vi "cDAQ Cal UI.vi"(11 "Calling VI Ref":refnum<vi>) -> ()   [LabVIEW 2013]
uses:
  Type Defs/Units Type Def (DAQ Rack).ctl
  Type Defs/cDAQ Type Def (cDAQ).ctl
  Type Defs/Rack Version Type Def.ctl
  Type Defs/Registered System.ctl
  Type Defs/System Type.ctl
  Type Defs/cDAQ Targets Type Def.ctl
  Type Defs/Target Cluster Type Def.ctl
  Type Defs/Setpoint Cluster Type Def.ctl
  Type Defs/TCP Data Stream Mode (PC).ctl
  <vilib>/Utility/miscctls.llb/LVRowAndColumnTypeDef.ctl
  <vilib>/Utility/file.llb/Write To Spreadsheet File (string).vi
  <vilib>/Utility/file.llb/Read From Spreadsheet File (string).vi
  <userlib>/_OpenG.lib/array/array.llb/Remove Duplicates from 1D Array (DBL)__ogtk.vi
  <userlib>/_OpenG.lib/array/array.llb/Search 1D Array (String)__ogtk.vi
  <vilib>/ptbypt/NI_PtbyPt.lvlib
  <vilib>/Analysis/NI_AALPro.lvlib
  <vilib>/Utility/config.llb/NI_LVConfig.lvlib
  <vilib>/FTP/NI_FTP.lvlib
panel:
  out "RIO Found":bool
  out "Lost Connection":bool
  in  "Stop Second Loop":bool
  out "a0":dbl format="%#.4g"
  out "a2":dbl format="%#.4g"
  out "a1":dbl format="%#.4g"
  out "a3":dbl format="%#.4g"
  out "a4":dbl format="%#.4g"
  in  "App Dir":path
  in  "Load Indicator Tab":enum32{"Page 1"}(tab)
  in  "Header Tab":enum32{"Page 1", "Page 2"}(tab)
  in  "Header OK":bool
  in  "Header Cancel":bool
  in  "Header Comments":string[][](table)=[[""], [""], [""]]
  in  "Cal Standards Table":string[][](table)=[["", ""], ["", ""], ["", ""], ["", ""], ["", ""]]
  in  "Sys Cal Table":string[][](table)=[["", ""], ["", ""], ["", ""], ["", ""], ["", ""]]
  in  "Header Table 1":string[][](table)=[[""], [""], [""], [""], [""], [""], [""], [""]]
  in  "Header Table 2":string[][](table)=[[""], [""], [""], [""], [""], [""], [""]]
  in  "debug":bool=TRUE
  in  "Output Tab":enum32{"Page 1", "Page 2"}(tab)
  out "Row":i32
  in  "Main Tab":enum32{"Page 1", "Page 2"}(tab)
  in  "Transfer Cal":bool
  in  "Verify Tab":enum32{"Page 1", "Page 2"}(tab)
  out "Ver Reading":dbl=0.0016 caption="reading" format="%#.4g"
  in  "Hide Devs":bool
  in  "Auto":bool
  in  "Hide Cal Values":bool
  in  "Verify Edit":bool
  in  "Verify Table":string[][](table)=[["", "0", "0"], ["", "3", "3"], ["", "6", "6"], ["", "9", "9"], ["", "12", "12"], ["", "15", "15"], ["", "", ""], ["", "", ""], ["", "", ""], ["", "", ""]]
  in  "Verify Read":bool
  in  "ms":u32=1000
  in  "avg":i32=5
  in  "Save Cal":bool
  in  "Cancel Verify":bool
  in  "Cal Tab":enum32{"Apply", "Cal"}(tab)
  in  "Cancel Cal":bool
  in  "Apply Cal":bool
  in  "Confirm Cal Point":bool
  in  "Master Value":dbl caption="cal pt" format="%#.4g"
  out "Cal Reading":dbl=0.0016 caption="reading" format="%#.4g"
  in  "4th Point Cal":bool
  out "Reading Value 4":dbl caption="reading" format="%#.4g"
  in  "Cal Value 4":dbl caption="cal pt" format="%#.4g"
  in  "5th Point Cal":bool
  out "Reading Value 5":dbl caption="reading" format="%#.4g"
  in  "Cal Value 5":dbl caption="cal pt" format="%#.4g"
  in  "Start Verification":bool
  in  "Header":bool
  out "Cal Table":string[][](table)=[["AI-00", "V", "", "", "", "", "", "", "", "", "", "", "", "", "", "", "", "", "", "", "", "", "", "", "", "", "", "", "", "", "", ""], ["AI-01", "V", "", "", "", "", "", "", "", "", "", "", "", "", "", "", "", "", "", "", "", "", "", "", "", "", "", "", "", "", "", ""], ["AI-02", "V", "", "", "", "", "", "", "", "", "", "", "", "", "", "", "", "", "", "", "", "", "", "", "", "", "", "", "", "", "", ""], ["AI-03", "V", "", "", "", "", "", "", "", "", "", "", "", "", "", "", "", "", "", "", "", "", "", "", "", "", "", "", "", "", "", ""], ["AI-04", "V", "", "", "", "", "", "", "", "", "", "", "", "", "", "", "", "", "", "", "", "", "", "", "", "", "", "", "", "", "", ""], ["AI-05", "V", "", "", "", "", "", "", "", "", "", "", "", "", "", "", "", "", "", "", "", "", "", "", "", "", "", "", "", "", "", ""], ["AI-06", "V", "", "", "", "", "", "", "", "", "", "", "", "", "", "", "", "", "", "", "", "", "", "", "", "", "", "", "", "", "", ""], ["AI-07", "V", "", "", "", "", "", "", "", "", "", "", "", "", "", "", "", "", "", "", "", "", "", "", "", "", "", "", "", "", "", ""], ["AI-08", "V", "", "", "", "", "", "", "", "", "", "", "", "", "", "", "", "", "", "", "", "", "", "", "", "", "", "", "", "", "", ""], ["AI-09", "V", "", "", "", "", "", "", "", "", "", "", "", "", "", "", "", "", "", "", "", "", "", "", "", "", "", "", "", "", "", ""], ["AI-10", "V", "", "", "", "", "", "", "", "", "", "", "", "", "", "", "", "", "", "", "", "", "", "", "", "", "", "", "", "", "", ""], ["AI-11", "V", "", "", "", "", "", "", "", "", "", "", "", "", "", "", "", "", "", "", "", "", "", "", "", "", "", "", "", "", "", ""], ["AI-12", "V", "", "", "", "", "", "", "", "", "", "", "", "", "", "", "", "", "", "", "", "", "", "", "", "", "", "", "", "", "", ""], ["AI-13", "V", "", "", "", "", "", "", "", "", "", "", "", "", "", "", "", "", "", "", "", "", "", "", "", "", "", "", "", "", "", ""], ["AI-14", "V", "", "", "", "", "", "", "", "", "", "", "", "", "", "", "", "", "", "", "", "", "", "", "", "", "", "", "", "", "", ""], ["AI-15", "V", "", "", "", "", "", "", "", "", "", "", "", "", "", "", "", "", "", "", "", "", "", "", "", "", "", "", "", "", "", ""], ["AI-16", "V", "", "", "", "", "", "", "", "", "", "", "", "", "", "", "", "", "", "", "", "", "", "", "", "", "", "", "", "", "", ""], ["AI-17", "V", "", "", "", "", "", "", "", "", "", "", "", "", "", "", "", "", "", "", "", "", "", "", "", "", "", "", "", "", "", ""], ["AI-18", "V", "", "", "", "", "", "", "", "", "", "", "", "", "", "", "", "", "", "", "", "", "", "", "", "", "", "", "", "", "", ""], ["AI-19", "V", "", "", "", "", "", "", "", "", "", "", "", "", "", "", "", "", "", "", "", "", "", "", "", "", "", "", "", "", "", ""], ["AI-20", "V", "", "", "", "", "", "", "", "", "", "", "", "", "", "", "", "", "", "", "", "", "", "", "", "", "", "", "", "", "", ""], ["AI-21", "V", "", "", "", "", "", "", "", "", "", "", "", "", "", "", "", "", "", "", "", "", "", "", "", "", "", "", "", "", "", ""], ["AI-22", "V", "", "", "", "", "", "", "", "", "", "", "", "", "", "", "", "", "", "", "", "", "", "", "", "", "", "", "", "", "", ""], ["AI-23", "V", "", "", "", "", "", "", "", "", "", "", "", "", "", "", "", "", "", "", "", "", "", "", "", "", "", "", "", "", "", ""], ["AI-24", "V", "", "", "", "", "", "", "", "", "", "", "", "", "", "", "", "", "", "", "", "", "", "", "", "", "", "", "", "", "", ""], ["AI-25", "V", "", "", "", "", "", "", "", "", "", "", "", "", "", "", "", "", "", "", "", "", "", "", "", "", "", "", "", "", "", ""], ["AI-26", "V", "", "", "", "", "", "", "", "", "", "", "", "", "", "", "", "", "", "", "", "", "", "", "", "", "", "", "", "", "", ""], ["AI-27", "V", "", "", "", "", "", "", "", "", "", "", "", "", "", "", "", "", "", "", "", "", "", "", "", "", "", "", "", "", "", ""], ["AI-28", "V", "", "", "", "", "", "", "", "", "", "", "", "", "", "", "", "", "", "", "", "", "", "", "", "", "", "", "", "", "", ""], ["AI-29", "V", "", "", "", "", "", "", "", "", "", "", "", "", "", "", "", "", "", "", "", "", "", "", "", "", "", "", "", "", "", ""], ["AI-30", "V", "", "", "", "", "", "", "", "", "", "", "", "", "", "", "", "", "", "", "", "", "", "", "", "", "", "", "", "", "", ""], ["AI-31", "V", "", "", "", "", "", "", "", "", "", "", "", "", "", "", "", "", "", "", "", "", "", "", "", "", "", "", "", "", "", ""], ["TC-00", "degF", "", "", "", "", "", "", "", "", "", "", "", "", "", "", "", "", "", "", "", "", "", "", "", "", "", "", "", "", "", ""], ["TC-01", "degF", "", "", "", "", "", "", "", "", "", "", "", "", "", "", "", "", "", "", "", "", "", "", "", "", "", "", "", "", "", ""], ["TC-02", "degF", "", "", "", "", "", "", "", "", "", "", "", "", "", "", "", "", "", "", "", "", "", "", "", "", "", "", "", "", "", ""], ["TC-03", "degF", "", "", "", "", "", "", "", "", "", "", "", "", "", "", "", "", "", "", "", "", "", "", "", "", "", "", "", "", "", ""], ["TC-04", "degF", "", "", "", "", "", "", "", "", "", "", "", "", "", "", "", "", "", "", "", "", "", "", "", "", "", "", "", "", "", ""], ["TC-05", "degF", "", "", "", "", "", "", "", "", "", "", "", "", "", "", "", "", "", "", "", "", "", "", "", "", "", "", "", "", "", ""], ["TC-06", "degF", "", "", "", "", "", "", "", "", "", "", "", "", "", "", "", "", "", "", "", "", "", "", "", "", "", "", "", "", "", ""], ["TC-07", "degF", "", "", "", "", "", "", "", "", "", "", "", "", "", "", "", "", "", "", "", "", "", "", "", "", "", "", "", "", "", ""], ["TC-08", "degF", "", "", "", "", "", "", "", "", "", "", "", "", "", "", "", "", "", "", "", "", "", "", "", "", "", "", "", "", "", ""], ["TC-09", "degF", "", "", "", "", "", "", "", "", "", "", "", "", "", "", "", "", "", "", "", "", "", "", "", "", "", "", "", "", "", ""], ["TC-10", "degF", "", "", "", "", "", "", "", "", "", "", "", "", "", "", "", "", "", "", "", "", "", "", "", "", "", "", "", "", "", ""], ["TC-11", "degF", "", "", "", "", "", "", "", "", "", "", "", "", "", "", "", "", "", "", "", "", "", "", "", "", "", "", "", "", "", ""], ["TC-12", "degF", "", "", "", "", "", "", "", "", "", "", "", "", "", "", "", "", "", "", "", "", "", "", "", "", "", "", "", "", "", ""], ["TC-13", "degF", "", "", "", "", "", "", "", "", "", "", "", "", "", "", "", "", "", "", "", "", "", "", "", "", "", "", "", "", "", ""], ["TC-14", "degF", "", "", "", "", "", "", "", "", "", "", "", "", "", "", "", "", "", "", "", "", "", "", "", "", "", "", "", "", "", ""], ["TC-15", "degF", "", "", "", "", "", "", "", "", "", "", "", "", "", "", "", "", "", "", "", "", "", "", "", "", "", "", "", "", "", ""], ["", "", "", "", "", "", "", "", "", "", "", "", "", "", "", "", "", "", "", "", "", "", "", "", "", "", "", "", "", "", "", ""]]
  out "Tank IP:":string
  in  "Start Cal":bool
  in  "1st Point Cal":bool
  out "Reading Value 1":dbl caption="Read Data" format="%#.4g"
  in  "Cal Value 1":dbl caption="Cal Point" format="%#.4g"
  in  "2nd Point Cal":bool
  out "Reading Value 2":dbl caption="reading" format="%#.4g"
  in  "Cal Value 2":dbl caption="cal pt" format="%#.4g"
  in  "Cal Unit":T1
  in  "3rd Point Cal":bool
  out "Reading Value 3":dbl caption="reading" format="%#.4g"
  in  "Cal Value 3":dbl caption="cal pt" format="%#.4g"
  in  "View Spreadsheet":bool
  in  "Channel to Cal":T2
  # "Channel Data"
  # "System Calibration Components"
  # "Calibration Standards Used"
  # "Output Control"
  # "Enter Header Info"
  # "Calibration"
  # "Verification"
  # "Select Channel to Calibrate"
  # "Cal Spreadsheet"
  # "*Excel must be closed to return control to this app."
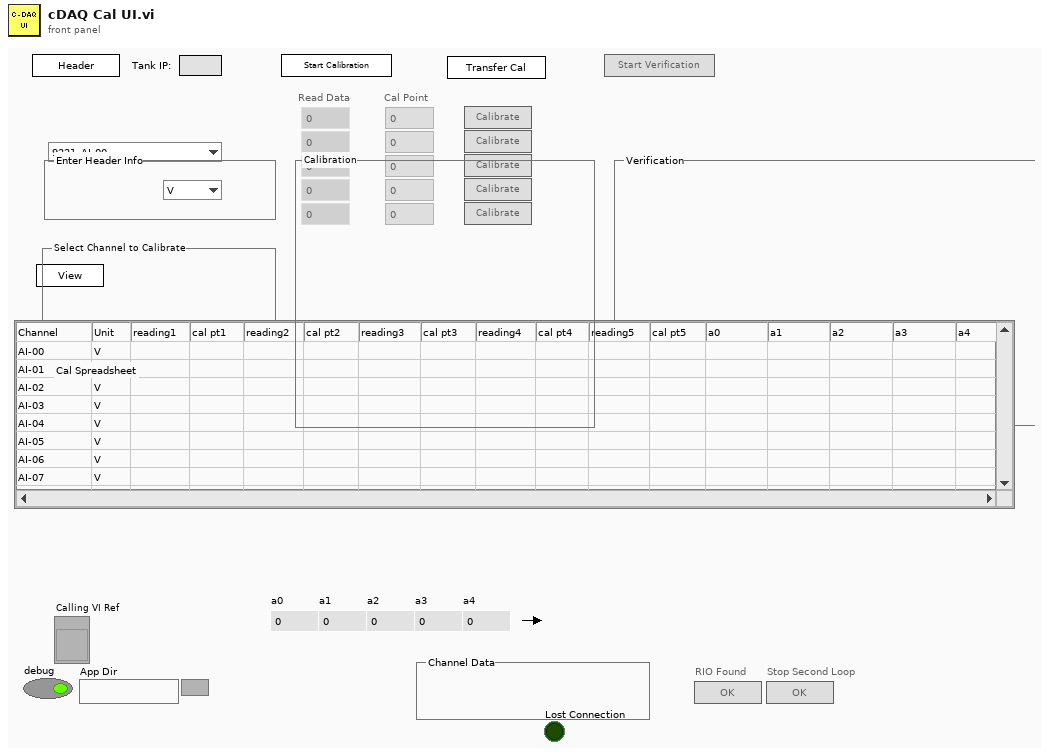
[diagram p1: front panel]
types:
  T1 = typedef "Units Type Def (DAQ Rack).ctl" = enum16{"V", "mA", "A", "Hz", "deg C"}
  T2 = typedef "cDAQ Type Def (cDAQ).ctl" = enum16{"9221_AI-00", "9221_AI-01", "9221_AI-02", "9221_AI-03", "9221_AI-04", "9221_AI-05", "9221_AI-06", "9221_AI-07", "9205_AI-00", "9205_AI-01", "9205_AI-02", "9205_AI-03", "9205_AI-04", "9205_AI-05", "9205_AI-06", "9205_AI-07", "9208_AI-00", "9208_AI-01", "9208_AI-02", "9208_AI-03", "9208_AI-04", "9208_AI-05", "9208_AI-06", "9208_AI-07", "9211_TC-00", "9211_TC-01", "9211_TC-02", "9211_TC-03"}
  T3 = typedef "cDAQ Targets Type Def.ctl" = cluster{"9221 Targets":T4, "9205 Targets":T4, "9208 Targets":T4, "9221 Setpoints":T5, "9205 Setpoints":T5, "9208 Setpoints ":T5, "9211 Targets":T4, "9211 Setpoints":T5}
  T4 = typedef "Target Cluster Type Def.ctl" = cluster{"target1":dbl, "target2":dbl, "target3":dbl, "target4":dbl, "target5":dbl, "target6":dbl, "target7":dbl, "target8":dbl, "target9":dbl, "target10":dbl}
  T5 = typedef "Setpoint Cluster Type Def.ctl" = cluster{"setpoint1":dbl, "setpoint2":dbl, "setpoint3":dbl, "setpoint4":dbl, "setpoint5":dbl}
  T6 = typedef "Registered System.ctl" = cluster{"System Type":T7, "Serial Number":string, "ID":string, "Cal File?":bool}
  T7 = typedef "System Type.ctl" = enum16{"DAQ Rack", "DAQ Cart", "RIO", "cDAQ", "unknown", "open"}
  T8 = typedef "Rack Version Type Def.ctl" = enum16{"Volts & TC", "Volts", "RIO", "cDAQ", "Volts & Current", "Cart"}
  T9 = cluster{"Error":errorcluster, "Cal Log":string[][], "Cal Log Header":string[], "Cal Files Base Path":path, "Default Cal Log":string[][], "Samples to Avg":i32, "Base Path":path, "Cal Targets Path":path, "Calling VI Ref":refnum<vi>, "Selected Chassis":tag, "debug":bool, "Verify Table":string[][], "Cal Template Path":path, "Cal Spreadsheet Path":path, "Verify Table Ref":refnum<vi>, "Init Mean":bool, "Auto":bool, "App Dir":path, "DAQ Rack":string, "Cal File Path":path, "cDAQ Targets":T3, "Cal Unit":T1, "Channel to Cal":T2, "Rack Version":T8, "Verification":bool, "Registered Systems":T6[], "Desired System":T6, "Cal Target Array":string[], "LastCalPt":i32, "StreamCtrlActive":bool}
  T10 = enum8{"Enabled", "Disabled", "Disabled and Grayed Out"}
  T11 = typedef "TCP Data Stream Mode (PC).ctl" = enum16{"Init", "Read Data", "Close"}
  T12 = typedef "LVRowAndColumnTypeDef.ctl" = cluster{"Row":i32, "Column":i32}
  T13 = enum32{"Bad", "Idle", "Run top level", "Running"}
  T14 = cluster{"[0]":dbl, "[1]":dbl, "[2]":dbl, "[3]":dbl, "[4]":dbl, "[5]":dbl, "[6]":dbl, "[7]":dbl, "[8]":dbl, "[9]":dbl}
  T15 = typedef "NI_LVConfig.lvlib/Config Data RefNum.ctl" = refnum<k1>
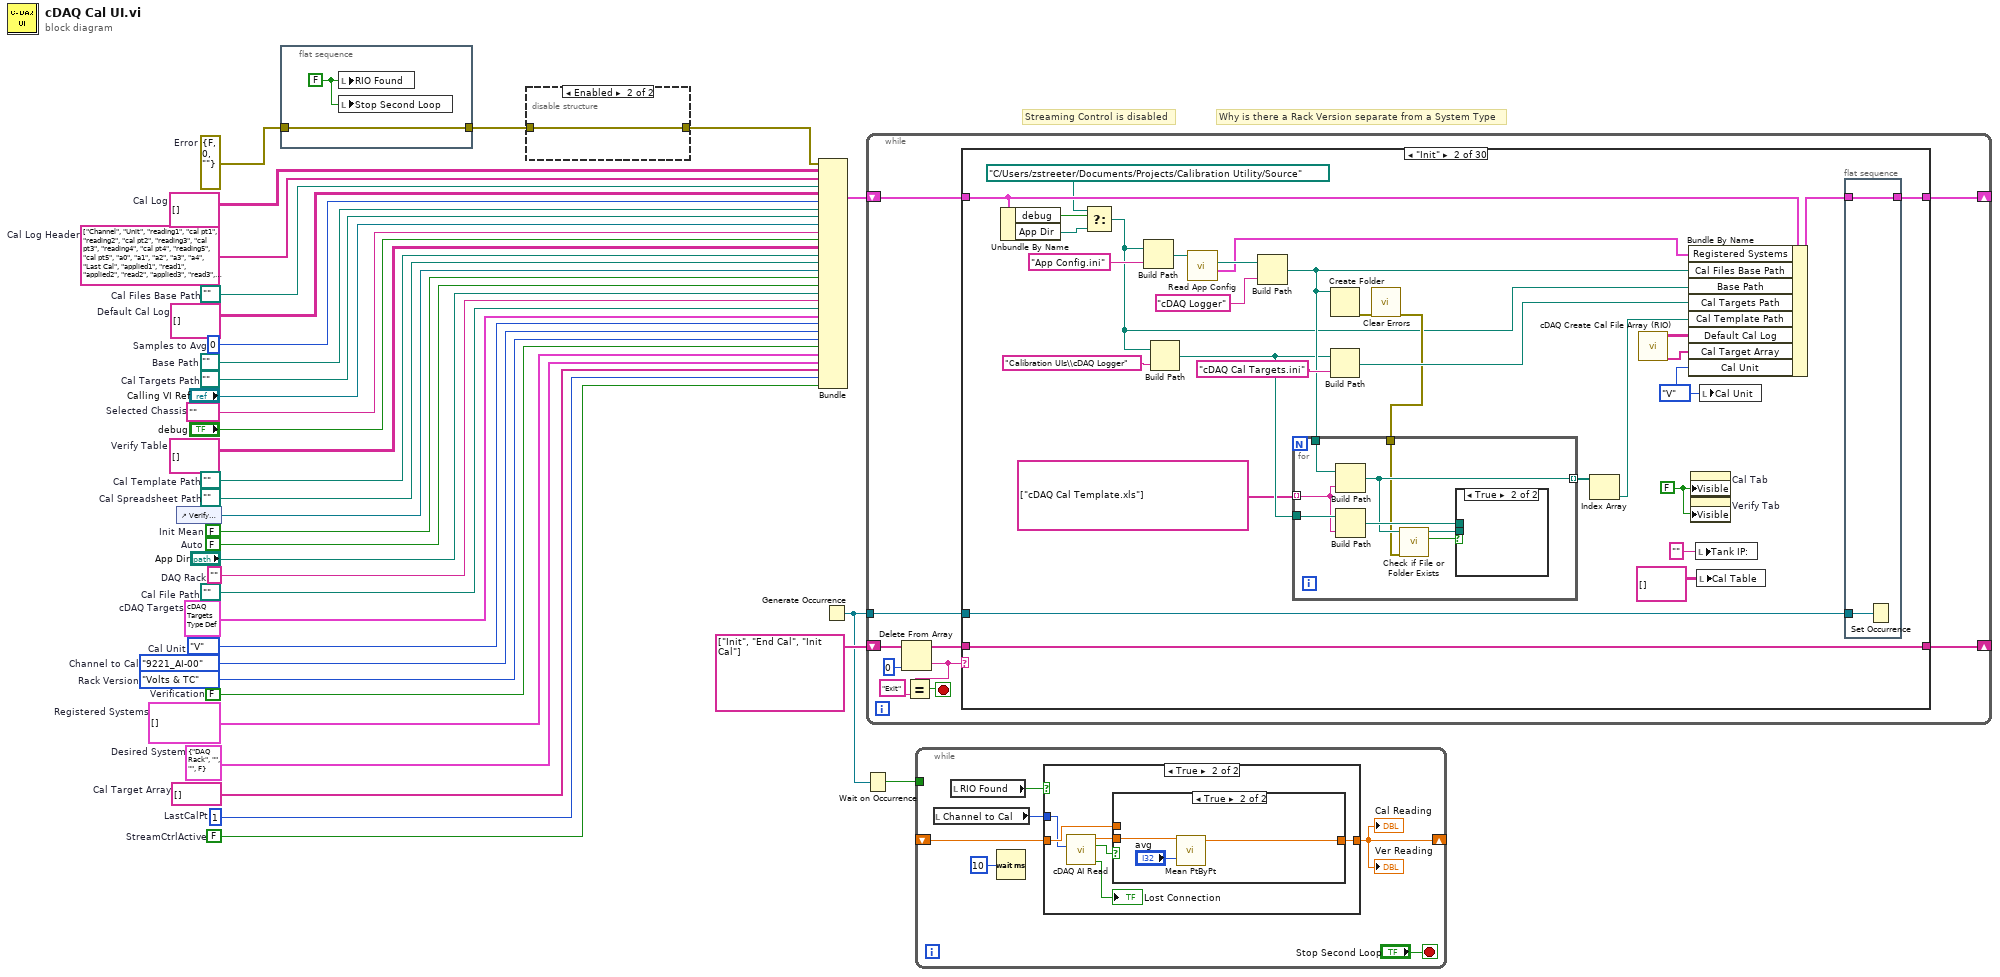
[diagram p0: block diagram]
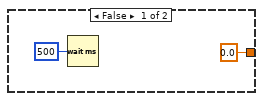
[diagram p2: hidden frame]
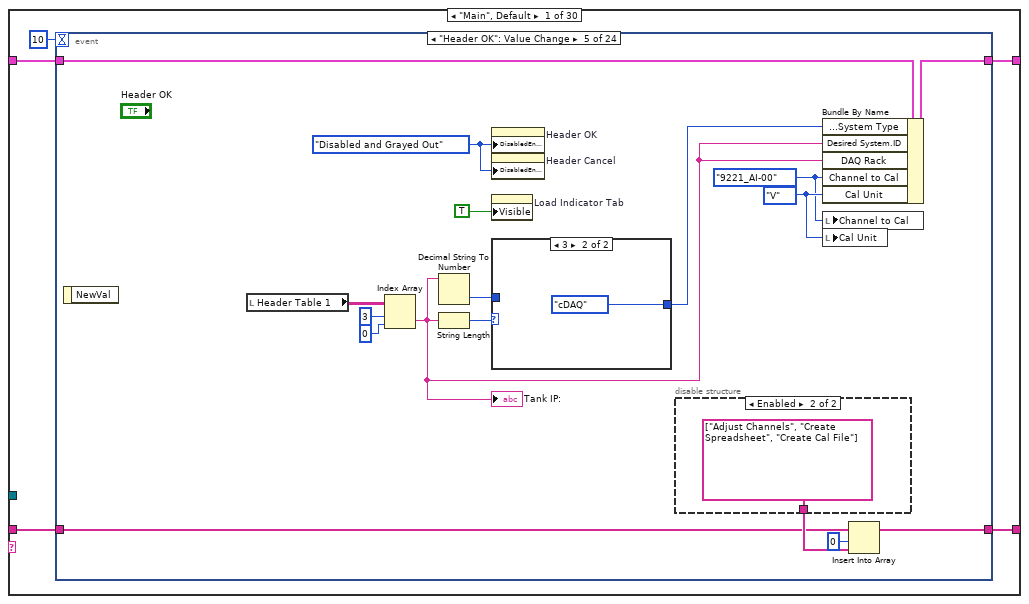
[diagram p4: hidden frame]
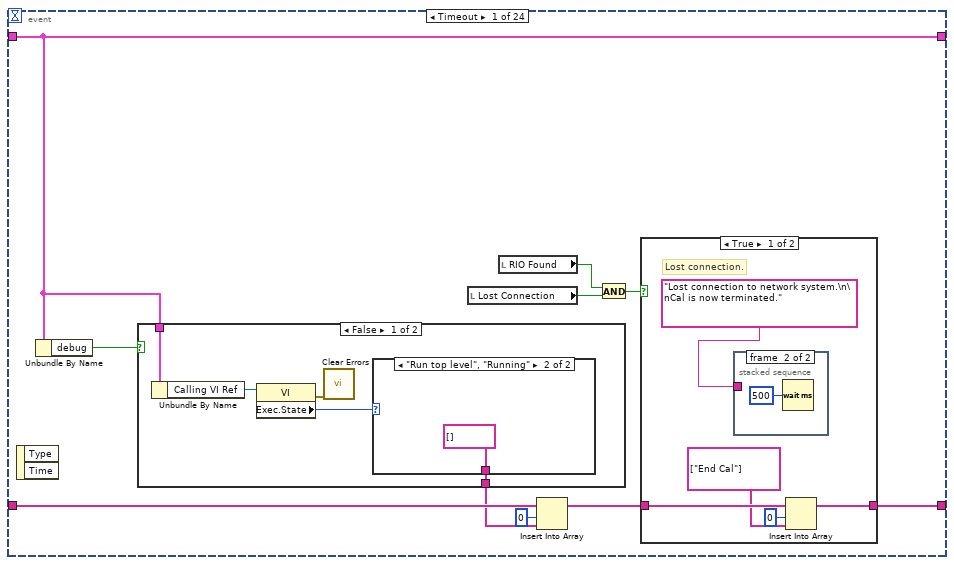
[diagram p5: hidden frame]
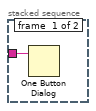
[diagram p6: hidden frame]
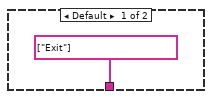
[diagram p8: hidden frame]
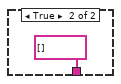
[diagram p9: hidden frame]
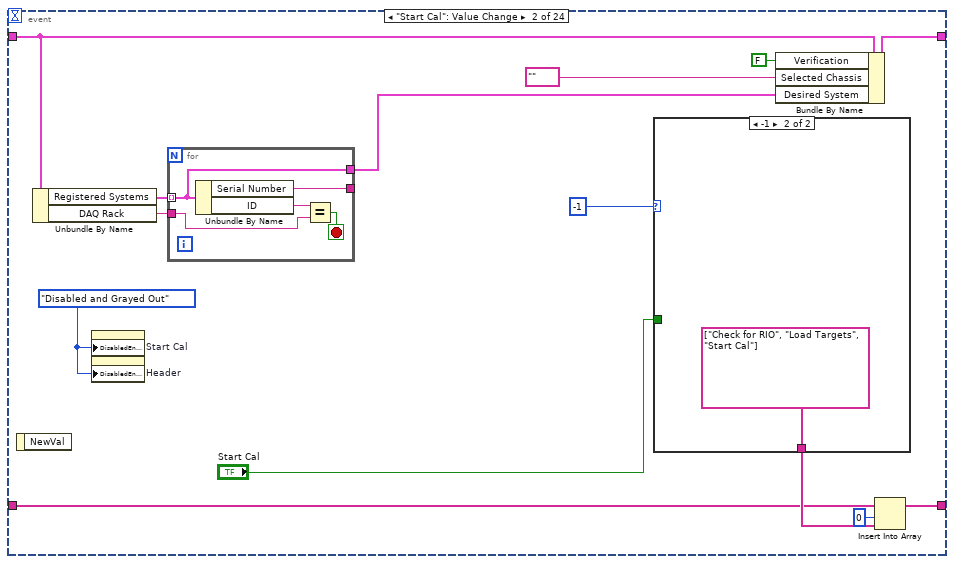
[diagram p10: hidden frame]
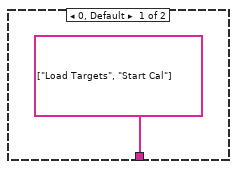
[diagram p11: hidden frame]
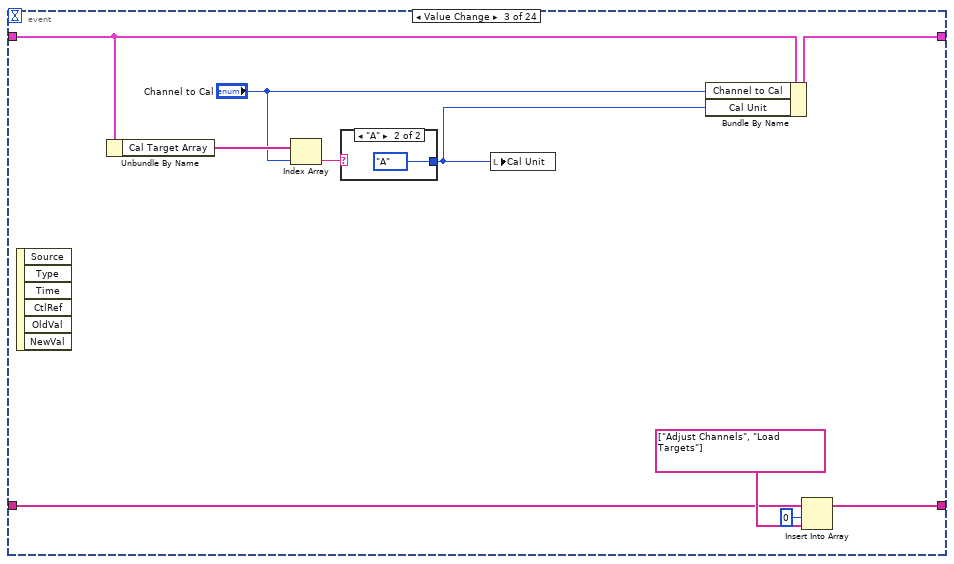
[diagram p12: hidden frame]
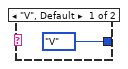
[diagram p13: hidden frame]
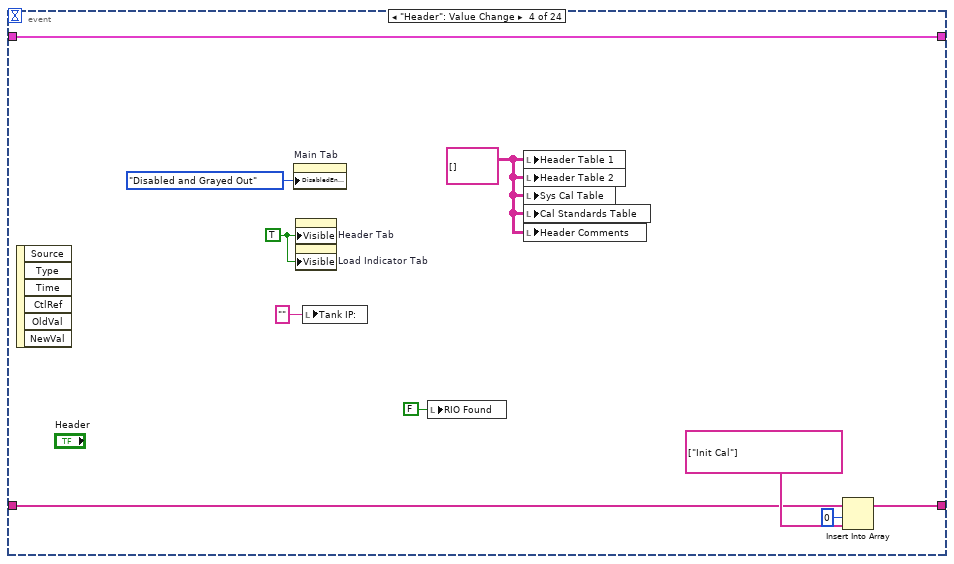
[diagram p14: hidden frame]
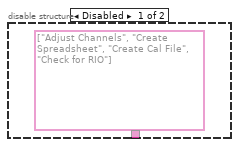
[diagram p15: hidden frame]
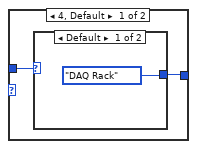
[diagram p16: hidden frame]
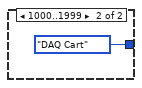
[diagram p17: hidden frame]
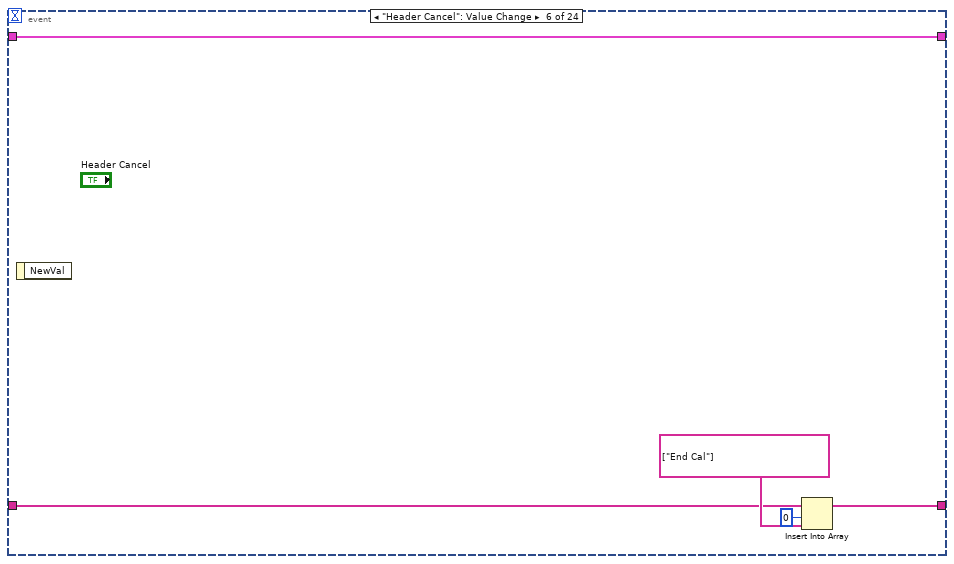
[diagram p18: hidden frame]
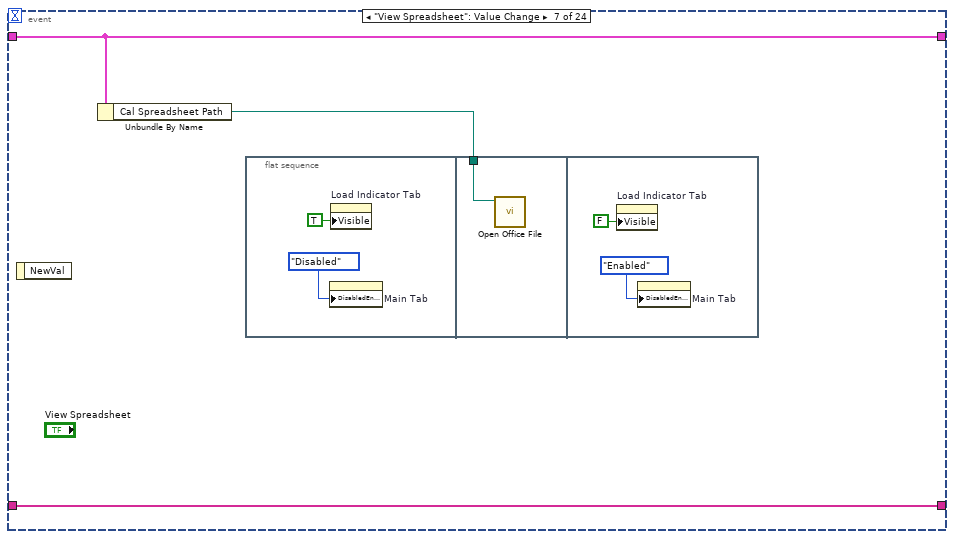
[diagram p19: hidden frame]
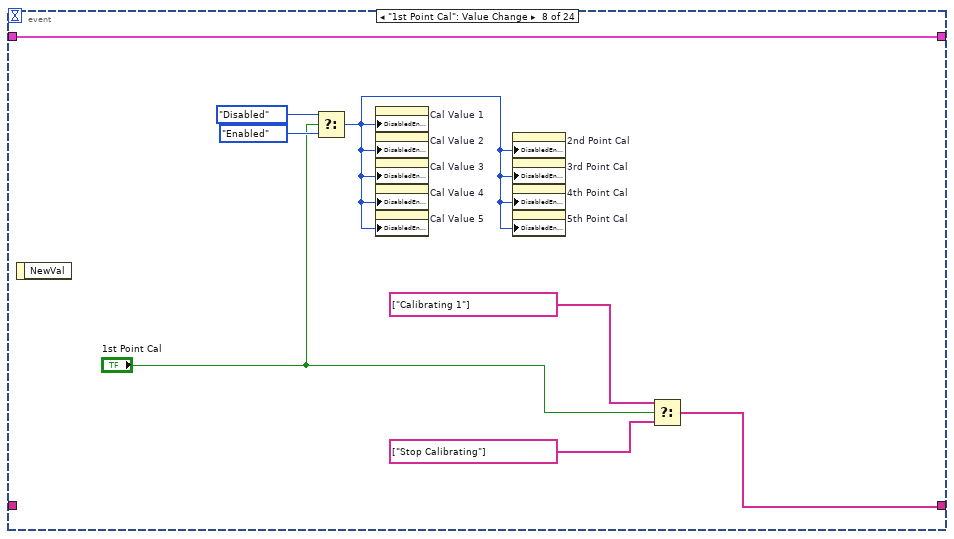
[diagram p20: hidden frame]
diagram:
  w1 = T3 {"9221 Targets"={"target1"=0.0, "target2"=0.0, "target3"=0.0, "target4"=0.0, "target5"=0.0, "target6"=0.0, "target7"=0.0, "target8"=0.0, "target9"=0.0, "target10"=0.0}, "9205 Targets"={"target1"=0.0, "target2"=0.0, "target3"=0.0, "target4"=0.0, "target5"=0.0, "target6"=0.0, "target7"=0.0, "target8"=0.0, "target9"=0.0, "target10"=0.0}, "9208 Targets"={"target1"=0.0, "target2"=0.0, "target3"=0.0, "target4"=0.0, "target5"=0.0, "target6"=0.0, "target7"=0.0, "target8"=0.0, "target9"=0.0, "target10"=0.0}, "9221 Setpoints"={"setpoint1"=0.0, "setpoint2"=0.0, "setpoint3"=0.0, "setpoint4"=0.0, "setpoint5"=0.0}, "9205 Setpoints"={"setpoint1"=0.0, "setpoint2"=0.0, "setpoint3"=0.0, "setpoint4"=0.0, "setpoint5"=0.0}, "9208 Setpoints "={"setpoint1"=0.0, "setpoint2"=0.0, "setpoint3"=0.0, "setpoint4"=0.0, "setpoint5"=0.0}, "9211 Targets"={"target1"=0.0, "target2"=0.0, "target3"=0.0, "target4"=0.0, "target5"=0.0, "target6"=0.0, "target7"=0.0, "target8"=0.0, "target9"=0.0, "target10"=0.0}, "9211 Setpoints"={"setpoint1"=0.0, "setpoint2"=0.0, "setpoint3"=0.0, "setpoint4"=0.0, "setpoint5"=0.0}}  # cDAQ Targets
  w2 = cDAQ_Type_Def_(cDAQ)."9221_AI-00"  # Channel to Cal
  w9 = FALSE  # StreamCtrlActive
  w10 = 1  # LastCalPt
  w12 = string[] ["Channel", "Unit", "reading1", "cal pt1", "reading2", "cal pt2", "reading3", "cal pt3", "reading4", "cal pt4", "reading5", "cal pt5", "a0", "a1", "a2", "a3", "a4", "Last Cal", "applied1", "read1", "applied2", "read2", "applied3", "read3", "applied4", "read4", "applied5", "read5", "applied6", "read6", "applied7", "read7", "applied8", "read8", "applied9", "read9", "applied10", "read10"]  # Cal Log Header
  w13 = string[] []  # Cal Target Array
  w14 = T6 {"System Type"=enum."DAQ Rack", "Serial Number"="", "ID"="", "Cal File?"=FALSE}  # Desired System
  w15 = T6[] []  # Registered Systems
  w16 = FALSE  # Verification
  w17 = Rack_Version_Type_Def."Volts & TC"  # Rack Version
  w18 = Units_Type_Def_(DAQ_Rack)."V"  # Cal Unit
  w19 = path ""  # Cal File Path
  w20 = ""  # DAQ Rack
  w22 = FALSE  # Auto
  w23 = FALSE  # Init Mean
  w25 = path ""  # Cal Spreadsheet Path
  w26 = path ""  # Cal Template Path
  w27 = string[][] []  # Verify Table
  w29 = tag ""  # Selected Chassis
  w31 = path ""  # Cal Targets Path
  w32 = path ""  # Base Path
  w33 = 0  # Samples to Avg
  w34 = string[][] []  # Default Cal Log
  w35 = path ""  # Cal Files Base Path
  w36 = string[][] []  # Cal Log
  w11 = errorcluster {"status"=FALSE, "code"=0, "source"=""}  # Error
  # "Why is there a Rack Version separate from a System Type"
  # "Streaming Control is disabled"
  n1 = control-ref of="Verify Table Ref"() -> (w24:refnum<vi>)
  n2 = flat-sequence {
    tunnel: w11 -> [w38]
    tunnel: [w38] -> w8
    frame #0 {
      w37 = FALSE ("RIO Found")
      n3 = local write "RIO Found"(w37) -> ()
      n4 = local write "Stop Second Loop"(w37) -> ()
    }
  }
  n5 = disable-structure shown="Enabled" {
    disable-tunnel: w8 -> [w42 w43]
    disable-tunnel: [w40 w43] -> w7
    frame Disabled {
      w39 = TRUE ("Visible")
      n6 = property on="Cal Tab" class="TabCtl (strict)"(error in=w42, "Visible"=w39) -> (error out=w41:errorcluster)  [unwired: 1 in, 1 out]
      n7 = property on="Verify Tab" class="TabCtl (strict)"(error in=w41, "Visible"=w39) -> (error out=w40:errorcluster)  [unwired: 1 in, 1 out]
    }
    frame Enabled {
    }
  }
  n8 = Bundle("Error"=w7, "Cal Log"=w36, "Cal Log Header"=w12, "Cal Files Base Path"=w35, "Default Cal Log"=w34, "Samples to Avg"=w33, "Base Path"=w32, "Cal Targets Path"=w31, "Calling VI Ref"="Calling VI Ref", "Selected Chassis"=w29, "debug"="debug", "Verify Table"=w27, "Cal Template Path"=w26, "Cal Spreadsheet Path"=w25, "Verify Table Ref"=w24, "Init Mean"=w23, "Auto"=w22, "App Dir"="App Dir", "DAQ Rack"=w20, "Cal File Path"=w19, "cDAQ Targets"=w1, "Cal Unit"=w18, "Channel to Cal"=w2, "Rack Version"=w17, "Verification"=w16, "Registered Systems"=w15, "Desired System"=w14, "Cal Target Array"=w13, "LastCalPt"=w10, "StreamCtrlActive"=w9) -> (w5:T9)  [unwired: 1 in]
  n9 = Generate Occurrence() -> (w4:refnum<k4>)
  n10 = Wait on Occurrence(2:w4) -> (0:w3:bool)  [unwired: 2 in]
  n11 = while {
    shift-right: [w46] -> _
    shift-left: string[] ["Init", "End Cal", "Init Cal"] -> [w53]
    shift-right: [w48] -> _
    shift-left: w5 -> [w49]
    tunnel: w4 -> [w44]
    stop <- w52 stop-if-true
    n12 = Delete From Array(array=w53, index=0) -> (deleted portion=w45:string, array with subset deleted=w51:string[])  [unwired: 1 in]
    n13 = Equal?(x=w45, y="Exit" ("x")) -> (x = y?=w52:bool)
    n14 = case shown="\"Init\"" w45 {
      selector: w45 -> [_ _ _ _ _ _ _ _ _ _ _ _ _ _ _ w816 _ _ _ _ _ _ _ _ _ _ _ _ _ _]
      tunnel: w51 -> [w57 w410 w425 w433 w449 w499 w520 w523 w527 w558 w588 w617 w641 w692 w806 w818 w832 w848 w932 w959 w969 w1032 w1110 w1134 w1150 w1161 w1184 w1197 w1205 w1208]
      tunnel: w49 -> [w56 w403 w426 w439 w446 w498 w519 w522 w525 w561 w590 w611 w639 w740 w809 w813 w833 w842 w918 w943 w970 w993 w1071 w1133 w1148 w1159 w1181 w1194 w1203 w1207]
      tunnel: [w55 w388 w426 w438 w446 w497 w518 w522 w525 w560 w590 w610 w643 w749 w809 w812 w833 w842 w918 w938 w970 w993 w1071 w1133 w1147 w1159 w1181 w1194 w1204 w1207] -> w48
      tunnel: [w54 w410 w425 w430 w448 w499 w520 w523 w526 w559 w589 w618 w642 w691 w806 w818 w832 w849 w931 w960 w969 w1033 w1111 w1134 w1149 w1160 w1184 w1198 w1205 w1208] -> w46
      tunnel: w44 -> [_ w387 _ _ _ _ _ _ _ _ _ _ _ _ _ _ _ _ _ _ _ _ _ _ _ _ _ _ _ _]
      frame "Main", Default {
        n15 = event shown="[4] \"Header OK\": Value Change" {
          selector: _ -> [_ _ _ _ _ _ _ _ _ _ _ _ _ _ _ _ _ _ _ _ _ _ _ _]
          dyn-events: _ -> [_ _ _ _ _ _ _ _ _ _ _ _ _ _ _ _ _ _ _ _ _ _ _ _]
          timeout: 10 -> [_ _ _ _ _ _ _ _ _ _ _ _ _ _ _ _ _ _ _ _ _ _ _ _]
          tunnel: w57 -> [w68 w96 w112 w122 w140 w155 w159 _ _ _ _ _ _ w218 w243 _ w285 _ w304 w337 w343 w367 w374 w380]
          tunnel: [w66 w94 w115 w127 w134 w153 w157 w172 w180 w188 w196 w204 w207 w221 w245 w279 w283 w292 w305 w338 w341 w361 w376 w381] -> w55
          tunnel: w56 -> [w66 w95 w110 w127 w135 w153 w157 w172 w180 w188 w196 w204 w207 w223 w245 w279 w284 w293 w305 w338 w341 w361 w376 w382]
          tunnel: [w61 w97 w111 w121 w141 w154 w159 w169 w177 w185 w193 w201 string[] ["Stop Verification"] w219 w243 string[] ["Save Cal"] w285 string[] ["Calc Dev", "Cal Review"] w304 w336 w342 w367 w375 w380] -> w54
          event Timeout {
            n16 = event-data() -> ()  [unwired: 1 in, 2 out]
            n17 = Unbundle By Name(w66) -> ("debug"=w65:bool)
            n18 = case shown="False" w65 {
              tunnel: [w81 string[] []] -> w67
              tunnel: w66 -> [w78 _]
              frame False {
                n19 = Unbundle By Name(w78) -> ("Calling VI Ref"=w80:refnum<vi>)
                n20 = property class="VI"(reference=w80) -> (error out=w77:errorcluster, "Exec.State"=w79:T13)  [unwired: 1 in, 1 out]
                n21 = call <vilib>:"Clear Errors.vi"("error in (no error)"=w77) -> ()  [unwired: 6 in, 1 out]
                n22 = case shown="\"Run top level\", \"Running\"" w79 {
                  tunnel: [string[] ["Exit"] string[] []] -> w81
                  frame Default {
                  }
                  frame "Run top level", "Running" {
                  }
                }
              }
              frame True {
              }
            }
            n23 = local read "Lost Connection"() -> (w60:bool)
            n24 = local read "RIO Found"() -> (w63:bool)
            n25 = Insert Into Array(array=w68, index=0, new element=w67) -> (w62:string[])
            n26 = And(x=w63, y=w60) -> (x .and. y?=w59:bool)
            n27 = case shown="True" w59 {
              tunnel: w62 -> [w73 w76]
              tunnel: [w70 w76] -> w61
              frame True {
                # "Lost connection."
                n28 = stacked-sequence {
                  tunnel: "Lost connection to network system.\n\nCal is now terminated." ("message") -> [w74 _]
                  frame #0 {
                    n29 = One Button Dialog(message=w74) -> ()  [unwired: 1 in, 1 out]
                  }
                  frame #1 {
                    n30 = Wait (ms)(milliseconds to wait=u32 500) -> ()  [unwired: 1 out]
                  }
                }
                n31 = Insert Into Array(array=w73, index=0, new element=string[] ["End Cal"]) -> (w70:string[])
              }
              frame False {
                # "Or not yet connected"
                # "Still connected."
              }
            }
          }
          event "Start Cal": Value Change {
            w92 = T10."Disabled and Grayed Out" ("Disabled")
            n32 = event-data() -> ()  [unwired: 1 in, 1 out]
            n33 = Unbundle By Name(w95) -> ("Registered Systems"=w90:T6[], "DAQ Rack"=w89:string)
            n34 = property on="Start Cal" class="Bool"("DisabledEnum"=w92) -> ()  [unwired: 2 in, 2 out]
            n35 = property on="Header" class="Bool"("DisabledEnum"=w92) -> ()  [unwired: 2 in, 2 out]
            n36 = for {
              tunnel: w90 -> [w99] mode=indexing
              tunnel: w89 -> [w102]
              tunnel: [w100] -> _
              tunnel: [w99] -> w88
              stop <- w101 stop-if-true
              n37 = Unbundle By Name(w99) -> ("Serial Number"=w100:string, "ID"=w103:string)
              n38 = Equal?(x=w103, y=w102) -> (x = y?=w101:bool)
            }
            n39 = case shown="-1" -1 ("index of element") {
              tunnel: [string[] ["Load Targets", "Start Cal"] string[] ["Check for RIO", "Load Targets", "Start Cal"]] -> w98
              tunnel: "Start Cal" -> [_ _]
              frame 0, Default {
              }
              frame -1 {
              }
            }
            n40 = Bundle By Name(cluster=w95, "Verification"=FALSE, "Selected Chassis"=tag "", "Desired System"=w88) -> (w94:T9)
            n41 = Insert Into Array(array=w96, index=0, new element=w98) -> (w97:string[])
          }
          event Value Change {
            n42 = event-data() -> ()  [unwired: 1 in, 6 out]
            n43 = Unbundle By Name(w110) -> ("Cal Target Array"=w109:string[])
            n44 = Index Array(array=w109, index="Channel to Cal") -> (element=w108:string)
            n45 = case shown="\"A\"" w108 {
              tunnel: [Units_Type_Def_(DAQ_Rack)."V" ("Cal Unit") Units_Type_Def_(DAQ_Rack)."A" ("Cal Unit")] -> w107
              frame "V", Default {
              }
              frame "A" {
              }
            }
            n46 = local write "Cal Unit"(w107) -> ()
            n47 = Bundle By Name(cluster=w110, "Channel to Cal"="Channel to Cal", "Cal Unit"=w107) -> (w115:T9)
            n48 = Insert Into Array(array=w112, index=0, new element=string[] ["Adjust Channels", "Load Targets"]) -> (w111:string[])
          }
          event "Header": Value Change {
            w125 = string[][] [] ("Header Table 1")
            w124 = TRUE ("Visible")
            n49 = event-data() -> ()  [unwired: 1 in, 6 out]
            n50 = property on="Main Tab" class="TabCtl (strict)"("DisabledEnum"=T10."Disabled and Grayed Out" ("Disabled")) -> ()  [unwired: 2 in, 2 out]
            n51 = property on="Header Tab" class="TabCtl (strict)"("Visible"=w124) -> ()  [unwired: 2 in, 2 out]
            n52 = property on="Load Indicator Tab" class="TabCtl (strict)"("Visible"=w124) -> ()  [unwired: 2 in, 2 out]
            n53 = local write "Tank IP:"("" ("DAQ Rack")) -> ()
            n54 = local write "RIO Found"(FALSE ("RIO Found")) -> ()
            n55 = local write "Header Table 1"(w125) -> ()
            n56 = local write "Header Table 2"(w125) -> ()
            n57 = local write "Sys Cal Table"(w125) -> ()
            n58 = local write "Cal Standards Table"(w125) -> ()
            n59 = local write "Header Comments"(w125) -> ()
            n60 = Insert Into Array(array=w122, index=0, new element=string[] ["Init Cal"]) -> (w121:string[])
          }
          event "Header OK": Value Change {
            w128 = cDAQ_Type_Def_(cDAQ)."9221_AI-00" ("Channel to Cal3")
            w133 = Units_Type_Def_(DAQ_Rack)."V" ("Cal Unit")
            w144 = T10."Disabled and Grayed Out" ("Disabled")
            n61 = event-data() -> ()  [unwired: 1 in, 1 out]
            n62 = local read "Header Table 1"() -> (w138:string[][])
            n63 = Index Array(array=w138, index (row)=3, index (col)=0 ("disabled index (col)")) -> (element=w130:string)
            "Tank IP:" <- w130
            n64 = Decimal String To Number(string=w130) -> (number=w129:i32)  [unwired: 2 in, 1 out]
            n65 = String Length(string=w130) -> (length=w132:i32)
            n66 = property on="Header OK" class="Bool"("DisabledEnum"=w144) -> ()  [unwired: 2 in, 2 out]
            n67 = property on="Header Cancel" class="Bool"("DisabledEnum"=w144) -> ()  [unwired: 2 in, 2 out]
            n68 = property on="Load Indicator Tab" class="TabCtl (strict)"("Visible"=TRUE) -> ()  [unwired: 2 in, 2 out]
            n69 = case shown="3" w132 {
              tunnel: [w147 System_Type."cDAQ" ("Desired System.System Type")] -> w131
              tunnel: w129 -> [w148 _]
              frame 4, Default {
                n70 = case shown="Default" w148 {
                  tunnel: [System_Type."DAQ Rack" ("Desired System.System Type") System_Type."DAQ Cart" ("Desired System.System Type")] -> w147
                  frame Default {
                  }
                  frame 1000..1999 {
                  }
                }
              }
              frame 3 {
              }
            }
            n71 = disable-structure shown="Enabled" {
              disable-tunnel: [string[] ["Adjust Channels", "Create Spreadsheet", "Create Cal File", "Check for RIO"] string[] ["Adjust Channels", "Create Spreadsheet", "Create Cal File"]] -> w142
              frame Disabled {
              }
              frame Enabled {
              }
            }
            n72 = Bundle By Name(cluster=w135, "Desired System.System Type"=w131, "Desired System.ID"=w130, "DAQ Rack"=w130, "Channel to Cal"=w128, "Cal Unit"=w133) -> (w134:T9)
            n73 = local write "Channel to Cal"(w128) -> ()
            n74 = local write "Cal Unit"(w133) -> ()
            n75 = Insert Into Array(array=w140, index=0, new element=w142) -> (w141:string[])
          }
          event "Header Cancel": Value Change {
            n76 = event-data() -> ()  [unwired: 1 in, 1 out]
            n77 = Insert Into Array(array=w155, index=0, new element=string[] ["End Cal"]) -> (w154:string[])
          }
          event "View Spreadsheet": Value Change {
            n78 = event-data() -> ()  [unwired: 1 in, 1 out]
            n79 = Unbundle By Name(w157) -> ("Cal Spreadsheet Path"=w158:path)
            n80 = flat-sequence {
              tunnel: w158 -> [w162]
              frame #0 {
                n81 = property on="Main Tab" class="TabCtl (strict)"("DisabledEnum"=T10."Disabled" ("Disabled")) -> ()  [unwired: 2 in, 2 out]
                n82 = property on="Load Indicator Tab" class="TabCtl (strict)"("Visible"=TRUE) -> ()  [unwired: 2 in, 2 out]
              }
              frame #1 {
                n83 = call "Open Office File.vi"("Selection a Word (.doc, .docx), Excel (.xls, .xlsx), or Powerpoint (.ppt, .pptx) Document..."=w162) -> ()  [unwired: 10 in, 1 out]
              }
              frame #2 {
                n84 = property on="Load Indicator Tab" class="TabCtl (strict)"("Visible"=FALSE) -> ()  [unwired: 2 in, 2 out]
                n85 = property on="Main Tab" class="TabCtl (strict)"("DisabledEnum"=T10."Enabled" ("Disabled")) -> ()  [unwired: 2 in, 2 out]
              }
            }
          }
          event "1st Point Cal": Value Change {
            n86 = event-data() -> ()  [unwired: 1 in, 1 out]
            n87 = Select(t=T10."Disabled" ("Disabled"), s="1st Point Cal", f=T10."Enabled" ("Disabled")) -> (s? t:f=w168:T10)
            n88 = property on="Cal Value 1" class="DigNum (strict)"("DisabledEnum"=w168) -> ()  [unwired: 2 in, 2 out]
            n89 = property on="Cal Value 2" class="DigNum (strict)"("DisabledEnum"=w168) -> ()  [unwired: 2 in, 2 out]
            n90 = property on="Cal Value 3" class="DigNum (strict)"("DisabledEnum"=w168) -> ()  [unwired: 2 in, 2 out]
            n91 = property on="Cal Value 4" class="DigNum (strict)"("DisabledEnum"=w168) -> ()  [unwired: 2 in, 2 out]
            n92 = property on="Cal Value 5" class="DigNum (strict)"("DisabledEnum"=w168) -> ()  [unwired: 2 in, 2 out]
            n93 = property on="2nd Point Cal" class="Bool (strict)"("DisabledEnum"=w168) -> ()  [unwired: 2 in, 2 out]
            n94 = property on="3rd Point Cal" class="Bool (strict)"("DisabledEnum"=w168) -> ()  [unwired: 2 in, 2 out]
            n95 = property on="4th Point Cal" class="Bool (strict)"("DisabledEnum"=w168) -> ()  [unwired: 2 in, 2 out]
            n96 = property on="5th Point Cal" class="Bool (strict)"("DisabledEnum"=w168) -> ()  [unwired: 2 in, 2 out]
            n97 = Select(t=string[] ["Calibrating 1"], s="1st Point Cal", f=string[] ["Stop Calibrating"]) -> (s? t:f=w169:string[])
          }
          event "2nd Point Cal": Value Change {
            n98 = event-data() -> ()  [unwired: 1 in, 1 out]
            n99 = Select(t=T10."Disabled" ("Disabled"), s="2nd Point Cal", f=T10."Enabled" ("Disabled")) -> (s? t:f=w176:T10)
            n100 = property on="Cal Value 1" class="DigNum (strict)"("DisabledEnum"=w176) -> ()  [unwired: 2 in, 2 out]
            n101 = property on="Cal Value 2" class="DigNum (strict)"("DisabledEnum"=w176) -> ()  [unwired: 2 in, 2 out]
            n102 = property on="Cal Value 3" class="DigNum (strict)"("DisabledEnum"=w176) -> ()  [unwired: 2 in, 2 out]
            n103 = property on="Cal Value 4" class="DigNum (strict)"("DisabledEnum"=w176) -> ()  [unwired: 2 in, 2 out]
            n104 = property on="Cal Value 5" class="DigNum (strict)"("DisabledEnum"=w176) -> ()  [unwired: 2 in, 2 out]
            n105 = property on="1st Point Cal" class="Bool (strict)"("DisabledEnum"=w176) -> ()  [unwired: 2 in, 2 out]
            n106 = property on="3rd Point Cal" class="Bool (strict)"("DisabledEnum"=w176) -> ()  [unwired: 2 in, 2 out]
            n107 = property on="4th Point Cal" class="Bool (strict)"("DisabledEnum"=w176) -> ()  [unwired: 2 in, 2 out]
            n108 = property on="5th Point Cal" class="Bool (strict)"("DisabledEnum"=w176) -> ()  [unwired: 2 in, 2 out]
            n109 = Select(t=string[] ["Calibrating 2"], s="2nd Point Cal", f=string[] ["Stop Calibrating"]) -> (s? t:f=w177:string[])
          }
          event "3rd Point Cal": Value Change {
            n110 = event-data() -> ()  [unwired: 1 in, 1 out]
            n111 = Select(t=T10."Disabled" ("Disabled"), s="3rd Point Cal", f=T10."Enabled" ("Disabled")) -> (s? t:f=w184:T10)
            n112 = property on="Cal Value 1" class="DigNum (strict)"("DisabledEnum"=w184) -> ()  [unwired: 2 in, 2 out]
            n113 = property on="Cal Value 2" class="DigNum (strict)"("DisabledEnum"=w184) -> ()  [unwired: 2 in, 2 out]
            n114 = property on="Cal Value 3" class="DigNum (strict)"("DisabledEnum"=w184) -> ()  [unwired: 2 in, 2 out]
            n115 = property on="Cal Value 4" class="DigNum (strict)"("DisabledEnum"=w184) -> ()  [unwired: 2 in, 2 out]
            n116 = property on="Cal Value 5" class="DigNum (strict)"("DisabledEnum"=w184) -> ()  [unwired: 2 in, 2 out]
            n117 = property on="1st Point Cal" class="Bool (strict)"("DisabledEnum"=w184) -> ()  [unwired: 2 in, 2 out]
            n118 = property on="2nd Point Cal" class="Bool (strict)"("DisabledEnum"=w184) -> ()  [unwired: 2 in, 2 out]
            n119 = property on="4th Point Cal" class="Bool (strict)"("DisabledEnum"=w184) -> ()  [unwired: 2 in, 2 out]
            n120 = property on="5th Point Cal" class="Bool (strict)"("DisabledEnum"=w184) -> ()  [unwired: 2 in, 2 out]
            n121 = Select(t=string[] ["Calibrating 3"], s="3rd Point Cal", f=string[] ["Stop Calibrating"]) -> (s? t:f=w185:string[])
          }
          event "4th Point Cal": Value Change {
            n122 = event-data() -> ()  [unwired: 1 in, 6 out]
            n123 = Select(t=T10."Disabled" ("Disabled"), s="4th Point Cal", f=T10."Enabled" ("Disabled")) -> (s? t:f=w192:T10)
            n124 = property on="Cal Value 1" class="DigNum (strict)"("DisabledEnum"=w192) -> ()  [unwired: 2 in, 2 out]
            n125 = property on="Cal Value 2" class="DigNum (strict)"("DisabledEnum"=w192) -> ()  [unwired: 2 in, 2 out]
            n126 = property on="Cal Value 3" class="DigNum (strict)"("DisabledEnum"=w192) -> ()  [unwired: 2 in, 2 out]
            n127 = property on="Cal Value 4" class="DigNum (strict)"("DisabledEnum"=w192) -> ()  [unwired: 2 in, 2 out]
            n128 = property on="Cal Value 5" class="DigNum (strict)"("DisabledEnum"=w192) -> ()  [unwired: 2 in, 2 out]
            n129 = property on="1st Point Cal" class="Bool (strict)"("DisabledEnum"=w192) -> ()  [unwired: 2 in, 2 out]
            n130 = property on="2nd Point Cal" class="Bool (strict)"("DisabledEnum"=w192) -> ()  [unwired: 2 in, 2 out]
            n131 = property on="3rd Point Cal" class="Bool (strict)"("DisabledEnum"=w192) -> ()  [unwired: 2 in, 2 out]
            n132 = property on="5th Point Cal" class="Bool (strict)"("DisabledEnum"=w192) -> ()  [unwired: 2 in, 2 out]
            n133 = Select(t=string[] ["Calibrating 4"], s="4th Point Cal", f=string[] ["Stop Calibrating"]) -> (s? t:f=w193:string[])
          }
          event "5th Point Cal": Value Change {
            n134 = event-data() -> ()  [unwired: 1 in, 6 out]
            n135 = Select(t=T10."Disabled" ("Disabled"), s="5th Point Cal", f=T10."Enabled" ("Disabled")) -> (s? t:f=w200:T10)
            n136 = property on="Cal Value 1" class="DigNum (strict)"("DisabledEnum"=w200) -> ()  [unwired: 2 in, 2 out]
            n137 = property on="Cal Value 2" class="DigNum (strict)"("DisabledEnum"=w200) -> ()  [unwired: 2 in, 2 out]
            n138 = property on="Cal Value 3" class="DigNum (strict)"("DisabledEnum"=w200) -> ()  [unwired: 2 in, 2 out]
            n139 = property on="Cal Value 4" class="DigNum (strict)"("DisabledEnum"=w200) -> ()  [unwired: 2 in, 2 out]
            n140 = property on="Cal Value 5" class="DigNum (strict)"("DisabledEnum"=w200) -> ()  [unwired: 2 in, 2 out]
            n141 = property on="1st Point Cal" class="Bool (strict)"("DisabledEnum"=w200) -> ()  [unwired: 2 in, 2 out]
            n142 = property on="2nd Point Cal" class="Bool (strict)"("DisabledEnum"=w200) -> ()  [unwired: 2 in, 2 out]
            n143 = property on="3rd Point Cal" class="Bool (strict)"("DisabledEnum"=w200) -> ()  [unwired: 2 in, 2 out]
            n144 = property on="4th Point Cal" class="Bool (strict)"("DisabledEnum"=w200) -> ()  [unwired: 2 in, 2 out]
            n145 = Select(t=string[] ["Calibrating 5"], s="5th Point Cal", f=string[] ["Stop Calibrating"]) -> (s? t:f=w201:string[])
          }
          event "Cancel Verify": Value Change {
            n146 = event-data() -> ()  [unwired: 1 in, 1 out]
            n147 = Unbundle By Name(w207) -> ("StreamCtrlActive"=w205:bool, "Desired System.ID"=w206:string)
            n148 = case shown="True" w205 {
              tunnel: w206 -> [_ w209]
              frame False {
              }
              frame True {
                w210 = FALSE
                n149 = Format Into String(format string="ni.var.psp://10.30.189.%s/Streaming Control/StreamCalibrated", w209) -> (resulting string=w216:string, error out=w217:errorcluster)  [unwired: 2 in]
                n150 = shared-variable-open(w216, w217, w210) -> (w211:refnum<k21>, w214:errorcluster)  [unwired: 1 in]
                n151 = shared-variable-write(w211, w214, w210) -> (w212:refnum<k21>, w213:errorcluster)
                n152 = Close Variable Connection(8:w213, 11:w212) -> ()  [unwired: 1 out]
              }
            }
          }
          event "Verify Read": Value Change {
            n153 = event-data() -> ()  [unwired: 1 in, 1 out]
            n154 = case shown="True" "Verify Read" {
              tunnel: [FALSE ("Verify Read") FALSE ("Verify Read")] -> w224
              tunnel: w223 -> [_ _]
              tunnel: w223 -> [w228 w234]
              tunnel: [w228 w233] -> w222
              tunnel: [w226 string[] ["Calc Dev", "Cal Review"]] -> w219
              tunnel: w218 -> [w226 _]
              frame False {
              }
              frame True {
                n155 = local read "Ver Reading"() -> (w229:dbl)
                n156 = local read "Verify Table"() -> (w230:string[][])
                n157 = local read "Row"() -> (w237:i32)
                n158 = Number To Fractional String(number=w229) -> (F-format string=w236:string)  [unwired: 3 in]
                n159 = Replace Array Subset(array=w230, new element=w236, index (row)=w237, index (col)=1 ("disabled index (col)")) -> (w232:string[][])
                n160 = Increment(x=w237) -> (x+1=w241:i32)
                n161 = Bundle(w241, "disabled index (col)"=1) -> (w238:cluster{i32, "disabled index (col)":i32})  [unwired: 1 in]
                n162 = Bundle By Name(cluster=w234, "Verify Table"=w232) -> (w233:T9)
                n163 = property on="Verify Table" class="Tbl (strict)"("Key Focus"=TRUE, "EditPos"=w238, "Value"=w232) -> ()  [unwired: 2 in, 2 out]
              }
            }
            n164 = local write "Verify Read"(w224) -> ()
            n165 = Bundle By Name(cluster=w222, "Init Mean"=TRUE ("initialize")) -> (w221:T9)
          }
          event "Verify Edit": Value Change {
            n166 = event-data() -> ()  [unwired: 1 in, 1 out]
            n167 = case shown="False" "Verify Edit" {
              tunnel: w245 -> [w260 _]
              frame False {
                w261 = T10."Enabled" ("Disabled")
                n168 = local read "Verify Table"() -> (w259:string[][])
                n169 = Unbundle By Name(w260) -> ("cDAQ Targets"=w257:T3, "Cal Targets Path"=w258:path, "Cal Target Array"=w247:string[], "Channel to Cal"=w248:T2)
                n170 = Index Array(array=w259, index (col)=0 ("disabled index (col)")) -> (element=w251:string[])  [unwired: 1 in]
                n171 = Fract/Exp String To Number(string=w251) -> (number=w250:dbl[])  [unwired: 3 in, 1 out]
                n172 = Index Array(array=w247, index=w248) -> (element=w246:string)
                n173 = Array To Cluster(array=w250) -> (cluster=w249:T14)
                n174 = case shown="\"9211\"" w246 {
                  tunnel: w257 -> [w266 w269 w272 w275]
                  tunnel: [w265 w268 w271 w274] -> w256
                  tunnel: w249 -> [w264 w267 w270 w273]
                  frame "9221", Default {
                    n175 = Bundle By Name(cluster=w266, "9221 Targets"=w264) -> (w265:T3)
                  }
                  frame "9205" {
                    n176 = Bundle By Name(cluster=w269, "9205 Targets"=w267) -> (w268:T3)
                  }
                  frame "9208" {
                    n177 = Bundle By Name(cluster=w272, "9208 Targets"=w270) -> (w271:T3)
                  }
                  frame "9211" {
                    n178 = Bundle By Name(cluster=w275, "9211 Targets"=w273) -> (w274:T3)
                  }
                }
                n179 = call <vilib>:"Open Config Data.vi"("configuration file path"=w258) -> ("error out"=w255:errorcluster, "refnum"=w254:T15)  [unwired: 8 in, 1 out]
                n180 = call <userlib>:"Write INI Cluster__ogtk.vi"("error in (no error)"=w255, "INI Fomatted Cluster"=w256, "refnum"=w254) -> ("error out"=w253:errorcluster, "dup refnum"=w252:T15)  [unwired: 7 in]
                n181 = property on="Hide Cal Values" class="Bool"("Visible"=TRUE) -> ()  [unwired: 2 in, 2 out]
                n182 = call <vilib>:"Close Config Data.vi"("error in (no error)"=w253, "refnum"=w252) -> ()  [unwired: 8 in, 2 out]
                n183 = property on="Verify Read" class="Bool (strict)"("DisabledEnum"=w261) -> ()  [unwired: 2 in, 2 out]
                n184 = property on="Auto" class="Bool (strict)"("DisabledEnum"=w261) -> ()  [unwired: 2 in, 2 out]
              }
              frame True {
                w276 = T10."Disabled and Grayed Out" ("Disabled")
                n185 = property on="Verify Read" class="Bool (strict)"("DisabledEnum"=w276) -> ()  [unwired: 2 in, 2 out]
                n186 = property on="Auto" class="Bool (strict)"("DisabledEnum"=w276) -> ()  [unwired: 2 in, 2 out]
                n187 = property on="Hide Cal Values" class="Bool"("Visible"=FALSE) -> ()  [unwired: 2 in, 2 out]
              }
            }
          }
          event "Save Cal": Value Change {
            n188 = event-data() -> ()  [unwired: 1 in, 1 out]
            n189 = property on="Cal Table" class="Tbl (strict)"("DisabledEnum"=T10."Enabled" ("Disabled")) -> ()  [unwired: 2 in, 2 out]
            n190 = property on="Verify Tab" class="TabCtl (strict)"("Visible"=FALSE) -> ()  [unwired: 2 in, 2 out]
          }
          event "Auto": Value Change {
            n191 = event-data() -> ()  [unwired: 1 in, 1 out]
            n192 = case shown="True" "Auto" {
              frame False {
              }
              frame True {
                n193 = local read "Row"() -> (w286:i32)
                n194 = Bundle("Row"=w286, "disabled index (col)"=1) -> (w287:cluster{"Row":i32, "disabled index (col)":i32})  [unwired: 1 in]
                n195 = property on="Verify Table" class="Tbl (strict)"("Key Focus"=TRUE, "EditPos"=w287) -> ()  [unwired: 2 in, 2 out]
              }
            }
            n196 = Bundle By Name(cluster=w284, "Auto"="Auto") -> (w283:T9)
          }
          event "Verify Table": Value Change {
            n197 = event-data() -> ()  [unwired: 1 in, 1 out]
            n198 = Bundle By Name(cluster=w293, "Verify Table"="Verify Table") -> (w292:T9)
          }
          event "Confirm Cal Point": Value Change {
            w298 = T10."Enabled" ("Disabled")
            n199 = event-data() -> ()  [unwired: 1 in, 1 out]
            n200 = local read "Cal Reading"() -> (w302:dbl)
            n201 = Unbundle By Name(w305) -> ("LastCalPt"=w303:i32)
            n202 = flat-sequence {
              tunnel: w303 -> [w309]
              tunnel: w302 -> [w308]
              tunnel: FALSE -> [w307]
              tunnel: "Master Value" -> [w306]
              tunnel: [w325] -> w297
              frame #0 {
                n203 = case shown="0, Default" w309 {
                  tunnel: w308 -> [_ w310 w313 w316 w319 w322]
                  tunnel: w306 -> [_ w312 w315 w318 w321 w324]
                  tunnel: w307 -> [_ w311 w314 w317 w320 w323]
                  frame 0, Default {
                  }
                  frame 1 {
                    n204 = local write "Cal Value 1"(w312) -> ()
                    n205 = local write "1st Point Cal"(w311) -> ()
                    "Reading Value 1" <- w310
                  }
                  frame 2 {
                    n206 = local write "Cal Value 2"(w315) -> ()
                    n207 = local write "2nd Point Cal"(w314) -> ()
                    "Reading Value 2" <- w313
                  }
                  frame 3 {
                    n208 = local write "Cal Value 3"(w318) -> ()
                    n209 = local write "3rd Point Cal"(w317) -> ()
                    "Reading Value 3" <- w316
                  }
                  frame 4 {
                    n210 = local write "Cal Value 4"(w321) -> ()
                    n211 = local write "4th Point Cal"(w320) -> ()
                    "Reading Value 4" <- w319
                  }
                  frame 5 {
                    n212 = local write "Cal Value 5"(w324) -> ()
                    n213 = local write "5th Point Cal"(w323) -> ()
                    "Reading Value 5" <- w322
                  }
                }
              }
              frame #1 {
                n214 = local read "Reading Value 2"() -> (w330:dbl)
                n215 = local read "Reading Value 3"() -> (w331:dbl)
                n216 = local read "Reading Value 4"() -> (w332:dbl)
                n217 = local read "Reading Value 5"() -> (w333:dbl)
                n218 = Not Equal To 0?(x=w330) -> (x != 0?=w329:bool)
                n219 = Not Equal To 0?(x=w331) -> (x != 0?=w328:bool)
                n220 = Not Equal To 0?(x=w332) -> (x != 0?=w327:bool)
                n221 = Not Equal To 0?(x=w333) -> (x != 0?=w326:bool)
                n222 = Compound Arithmetic op=AND(w329, w328, w327, w326) -> (w325:bool)
              }
            }
            n223 = property on="Cal Value 1" class="DigNum (strict)"("DisabledEnum"=w298) -> ()  [unwired: 2 in, 2 out]
            n224 = property on="Cal Value 2" class="DigNum (strict)"("DisabledEnum"=w298) -> ()  [unwired: 2 in, 2 out]
            n225 = property on="Cal Value 3" class="DigNum (strict)"("DisabledEnum"=w298) -> ()  [unwired: 2 in, 2 out]
            n226 = property on="Cal Value 4" class="DigNum (strict)"("DisabledEnum"=w298) -> ()  [unwired: 2 in, 2 out]
            n227 = property on="Cal Value 5" class="DigNum (strict)"("DisabledEnum"=w298) -> ()  [unwired: 2 in, 2 out]
            n228 = property on="1st Point Cal" class="Bool (strict)"("DisabledEnum"=w298) -> ()  [unwired: 2 in, 2 out]
            n229 = property on="2nd Point Cal" class="Bool (strict)"("DisabledEnum"=w298) -> ()  [unwired: 2 in, 2 out]
            n230 = property on="3rd Point Cal" class="Bool (strict)"("DisabledEnum"=w298) -> ()  [unwired: 2 in, 2 out]
            n231 = property on="4th Point Cal" class="Bool (strict)"("DisabledEnum"=w298) -> ()  [unwired: 2 in, 2 out]
            n232 = property on="5th Point Cal" class="Bool (strict)"("DisabledEnum"=w298) -> ()  [unwired: 2 in, 2 out]
            n233 = local write "Cal Tab"(enum32{"Apply", "Cal"}."Apply" ("Cal Tab")) -> ()
            n234 = Select(t=T10."Enabled" ("Disabled"), s=w297, f=T10."Disabled and Grayed Out" ("Disabled")) -> (s? t:f=w294:T10)
            n235 = property on="Apply Cal" class="Bool"("DisabledEnum"=w294) -> ()  [unwired: 2 in, 2 out]
          }
          event "Apply Cal": Value Change {
            n236 = event-data() -> ()  [unwired: 1 in, 6 out]
            n237 = Insert Into Array(array=w337, index=0, new element=string[] ["Calculate Coeffs"]) -> (w336:string[])
          }
          event "Start Verification": Value Change {
            n238 = event-data() -> ()  [unwired: 1 in, 6 out]
            n239 = Unbundle By Name(w341) -> ("StreamCtrlActive"=w339:bool, "Desired System.ID"=w340:string)
            n240 = case shown="True" w339 {
              tunnel: w340 -> [_ w347]
              frame False {
              }
              frame True {
                n241 = Format Into String(format string="ni.var.psp://10.30.189.%s/Streaming Control/StreamCalibrated", w347) -> (resulting string=w355:string, error out=w356:errorcluster)  [unwired: 2 in]
                n242 = shared-variable-open(w355, w356, FALSE) -> (w349:refnum<k21>, w352:errorcluster)  [unwired: 1 in]
                n243 = shared-variable-write(w349, w352, TRUE ("data in")) -> (w350:refnum<k21>, w351:errorcluster)
                n244 = Close Variable Connection(8:w351, 11:w350) -> ()  [unwired: 1 out]
              }
            }
            n245 = property on="Verify Tab" class="TabCtl (strict)"("Visible"="Start Verification") -> ()  [unwired: 2 in, 2 out]
            n246 = Insert Into Array(array=w343, index=0, new element=string[] ["Load Targets", "Calculate Coeffs"]) -> (w342:string[])
          }
          event "Cancel Cal": Value Change {
            w368 = T10."Disabled and Grayed Out" ("Disabled")
            w358 = T10."Enabled" ("Disabled")
            n247 = event-data() -> ()  [unwired: 1 in, 6 out]
            n248 = Unbundle By Name(w361) -> ("Desired System.ID"=w364:string)
            n249 = Format Into String(format string="192.168.1.%s", w364) -> (resulting string=w360:string)  [unwired: 2 in, 1 out]
            n250 = flat-sequence {
              tunnel: w360 -> [w370]
              tunnel: [w370] -> w362
              tunnel: [w373] -> w359
              tunnel: w362 -> [w373]
              frame #0 {
                n251 = local write "RIO Found"(FALSE ("RIO Found")) -> ()
              }
              frame #1 {
                n252 = Wait (ms)(milliseconds to wait=u32 20) -> ()  [unwired: 1 out]
              }
            }
            n253 = property on="Cal Tab" class="TabCtl (strict)"("Visible"=FALSE) -> ()  [unwired: 2 in, 2 out]
            n254 = property on="Cal Unit" class="Enum (strict)"("DisabledEnum"=T10."Enabled" ("Disabled")) -> ()  [unwired: 2 in, 2 out]
            n255 = property on="Header" class="Bool"("DisabledEnum"=w358) -> ()  [unwired: 2 in, 2 out]
            n256 = property on="Channel to Cal" class="Enum (strict)"("DisabledEnum"=w358) -> ()  [unwired: 2 in, 2 out]
            n257 = property on="View Spreadsheet" class="Bool"("DisabledEnum"=w358) -> ()  [unwired: 2 in, 2 out]
            n258 = property on="Start Cal" class="Bool"("DisabledEnum"=w358) -> ()  [unwired: 2 in, 2 out]
            n259 = call "TCP Data Stream PC.vi"("RT IP Address"=w359, "Mode"=TCP_Data_Stream_Mode_(PC)."Close") -> ()  [unwired: 14 in, 4 out]
            n260 = disable-structure shown="Disabled" {
              disable-tunnel: w358 -> [w369 _]
              frame Disabled {
                n261 = property on="Start Verification" class="Bool"("DisabledEnum"=w369) -> ()  [unwired: 2 in, 2 out]
              }
              frame Enabled {
              }
            }
            n262 = property on="Reading Value 1" class="DigNum (strict)"("DisabledEnum"=w368) -> ()  [unwired: 2 in, 2 out]
            n263 = property on="Cal Value 1" class="DigNum (strict)"("DisabledEnum"=w368) -> ()  [unwired: 2 in, 2 out]
            n264 = property on="1st Point Cal" class="Bool (strict)"("DisabledEnum"=w368) -> ()  [unwired: 2 in, 2 out]
            n265 = property on="Reading Value 2" class="DigNum (strict)"("DisabledEnum"=w368) -> ()  [unwired: 2 in, 2 out]
            n266 = property on="Cal Value 2" class="DigNum (strict)"("DisabledEnum"=w368) -> ()  [unwired: 2 in, 2 out]
            n267 = property on="2nd Point Cal" class="Bool (strict)"("DisabledEnum"=w368) -> ()  [unwired: 2 in, 2 out]
            n268 = property on="Reading Value 3" class="DigNum (strict)"("DisabledEnum"=w368) -> ()  [unwired: 2 in, 2 out]
            n269 = property on="Cal Value 3" class="DigNum (strict)"("DisabledEnum"=w368) -> ()  [unwired: 2 in, 2 out]
            n270 = property on="3rd Point Cal" class="Bool (strict)"("DisabledEnum"=w368) -> ()  [unwired: 2 in, 2 out]
            n271 = property on="Reading Value 4" class="DigNum (strict)"("DisabledEnum"=w368) -> ()  [unwired: 2 in, 2 out]
            n272 = property on="Cal Value 4" class="DigNum (strict)"("DisabledEnum"=w368) -> ()  [unwired: 2 in, 2 out]
            n273 = property on="4th Point Cal" class="Bool (strict)"("DisabledEnum"=w368) -> ()  [unwired: 2 in, 2 out]
            n274 = property on="Reading Value 5" class="DigNum (strict)"("DisabledEnum"=w368) -> ()  [unwired: 2 in, 2 out]
            n275 = property on="Cal Value 5" class="DigNum (strict)"("DisabledEnum"=w368) -> ()  [unwired: 2 in, 2 out]
            n276 = property on="5th Point Cal" class="Bool (strict)"("DisabledEnum"=w368) -> ()  [unwired: 2 in, 2 out]
          }
          event "Transfer Cal": Value Change {
            n277 = event-data() -> ()  [unwired: 1 in, 6 out]
            n278 = disable-structure shown="Disabled" {
              disable-tunnel: [string[] ["Distribute Calibration"] w378] -> w375
              disable-tunnel: w374 -> [_ w378]
              frame Disabled {
              }
              frame Enabled {
              }
            }
          }
          event Value Change {
            n279 = event-data() -> ()  [unwired: 1 in, 1 out]
            n280 = Bundle By Name(cluster=w382, "Cal Unit"="Cal Unit") -> (w381:T9)
          }
        }
      }
      frame "Init" {
        w390 = FALSE ("Visible")
        w395 = Units_Type_Def_(DAQ_Rack)."V" ("Cal Unit")
        n281 = Unbundle By Name(w403) -> ("debug"=w402:bool, "App Dir"=w401:path)
        n282 = Select(t=path "C:/Users/zstreeter/Documents/Projects/Calibration Utility/Source", s=w402, f=w401) -> (s? t:f=w400:path)
        n283 = Build Path(base path=w400, name or relative path="App Config.ini") -> (appended path=w406:path)
        n284 = Build Path(base path=w400, name or relative path="Calibration UIs\\cDAQ Logger") -> (appended path=w398:path)
        n285 = call "Read App Config.vi"("App Config Path"=w406) -> ("Registered cDAQ Systems"=w383:T6[], "Cal Files Path"=w409:path)  [unwired: 8 in, 1 out]
        n286 = Build Path(base path=w409, name or relative path="cDAQ Logger") -> (appended path=w405:path)
        n287 = Create Folder(path (use dialog)=w405) -> (error out=w411:errorcluster)  [unwired: 2 in, 2 out]
        n288 = Build Path(base path=w398, name or relative path="cDAQ Cal Targets.ini") -> (appended path=w408:path)
        n289 = call <vilib>:"Clear Errors.vi"("error in (no error)"=w411) -> ("error out"=w404:errorcluster)  [unwired: 6 in]
        n290 = for {
          tunnel: [w419] -> w397 mode=indexing
          tunnel: w405 -> [w418]
          tunnel: w404 -> [w417]
          tunnel: w398 -> [w416]
          tunnel: string[] ["cDAQ Cal Template.xls"] -> [w415] mode=indexing
          n291 = Build Path(base path=w418, name or relative path=w415) -> (appended path=w419:path)
          n292 = Build Path(base path=w416, name or relative path=w415) -> (appended path=w422:path)
          n293 = call <vilib>:"Check if File or Folder Exists.vi"("error in (no error)"=w417, "path"=w419) -> ("file or folder exists?"=w420:bool, "dup path"=w421:path)  [unwired: 7 in, 1 out]
          n294 = case shown="True" w420 {
            tunnel: w421 -> [w424 _]
            tunnel: w422 -> [w423 _]
            frame False {
              n295 = Copy(10:w424, 11:w423) -> ()  [unwired: 3 in, 3 out]
            }
            frame True {
            }
          }
        }
        n296 = Index Array(array=w397) -> (element=w394:path)  [unwired: 1 in]
        n297 = call "cDAQ Create Cal File Array (RIO).vi"() -> ("Cal Target Array"=w384:string[], "Cal Log OUT"=w385:string[][])  [unwired: 10 in]
        n298 = Bundle By Name(cluster=w403, "Registered Systems"=w383, "Cal Files Base Path"=w405, "Base Path"=w400, "Cal Targets Path"=w408, "Cal Template Path"=w394, "Default Cal Log"=w385, "Cal Target Array"=w384, "Cal Unit"=w395) -> (w389:T9)
        n299 = property on="Cal Tab" class="TabCtl (strict)"("Visible"=w390) -> ()  [unwired: 2 in, 2 out]
        n300 = property on="Verify Tab" class="TabCtl (strict)"("Visible"=w390) -> ()  [unwired: 2 in, 2 out]
        n301 = local write "Tank IP:"("" ("DAQ Rack")) -> ()
        n302 = local write "Cal Table"(string[][] []) -> ()
        n303 = local write "Cal Unit"(w395) -> ()
        n304 = flat-sequence {
          tunnel: w389 -> [w414]
          tunnel: [w414] -> w388
          tunnel: w387 -> [w413]
          frame #0 {
            n305 = Set Occurrence(w413) -> ()
          }
        }
      }
      frame "Unused Items" {
      }
      frame "Init Cal" {
        w429 = FALSE ("Auto")
        w435 = FALSE ("Verify Read")
        w436 = T10."Enabled" ("Disabled")
        w428 = FALSE ("Visible")
        w427 = T10."Disabled and Grayed Out" ("Disabled")
        n306 = Unbundle By Name(w439) -> ("Cal Log Header"=w431:string[])
        n307 = property on="Cal Table" class="Tbl (strict)"("Column Headers[]"=w431) -> ()  [unwired: 2 in, 2 out]
        n308 = property on="Reading Value 1" class="DigNum (strict)"("DisabledEnum"=w427) -> ()  [unwired: 2 in, 2 out]
        n309 = property on="Cal Value 1" class="DigNum (strict)"("DisabledEnum"=w427) -> ()  [unwired: 2 in, 2 out]
        n310 = property on="1st Point Cal" class="Bool (strict)"("DisabledEnum"=w427) -> ()  [unwired: 2 in, 2 out]
        n311 = property on="Reading Value 2" class="DigNum (strict)"("DisabledEnum"=w427) -> ()  [unwired: 2 in, 2 out]
        n312 = property on="Cal Value 2" class="DigNum (strict)"("DisabledEnum"=w427) -> ()  [unwired: 2 in, 2 out]
        n313 = property on="2nd Point Cal" class="Bool (strict)"("DisabledEnum"=w427) -> ()  [unwired: 2 in, 2 out]
        n314 = property on="Reading Value 3" class="DigNum (strict)"("DisabledEnum"=w427) -> ()  [unwired: 2 in, 2 out]
        n315 = property on="Cal Value 3" class="DigNum (strict)"("DisabledEnum"=w427) -> ()  [unwired: 2 in, 2 out]
        n316 = property on="3rd Point Cal" class="Bool (strict)"("DisabledEnum"=w427) -> ()  [unwired: 2 in, 2 out]
        n317 = property on="Reading Value 4" class="DigNum (strict)"("DisabledEnum"=w427) -> ()  [unwired: 2 in, 2 out]
        n318 = property on="Cal Value 4" class="DigNum (strict)"("DisabledEnum"=w427) -> ()  [unwired: 2 in, 2 out]
        n319 = property on="4th Point Cal" class="Bool (strict)"("DisabledEnum"=w427) -> ()  [unwired: 2 in, 2 out]
        n320 = property on="Reading Value 5" class="DigNum (strict)"("DisabledEnum"=w427) -> ()  [unwired: 2 in, 2 out]
        n321 = property on="Cal Value 5" class="DigNum (strict)"("DisabledEnum"=w427) -> ()  [unwired: 2 in, 2 out]
        n322 = property on="5th Point Cal" class="Bool (strict)"("DisabledEnum"=w427) -> ()  [unwired: 2 in, 2 out]
        n323 = property on="Verify Read" class="Bool (strict)"("DisabledEnum"=w436) -> ()  [unwired: 2 in, 2 out]
        n324 = property on="Cal Table" class="Tbl (strict)"("DisabledEnum"=w436) -> ()  [unwired: 2 in, 2 out]
        n325 = property on="Verify Tab" class="TabCtl (strict)"("Visible"=w428) -> ()  [unwired: 2 in, 2 out]
        n326 = property on="Cal Tab" class="TabCtl (strict)"("Visible"=w428) -> ()  [unwired: 2 in, 2 out]
        n327 = property on="Hide Cal Values" class="Bool"("Visible"=TRUE) -> ()  [unwired: 2 in, 2 out]
        n328 = local write "Verify Read"(w435) -> ()
        n329 = local write "Auto"(w435) -> ()
        n330 = local write "Verify Edit"(w435) -> ()
        n331 = Bundle By Name(cluster=w439, "Auto"=w429, "Verification"=w429) -> (w438:T9)
        n332 = Insert Into Array(array=w433, index=0, new element=string[] ["Clear Dev Data", "Update Dev Tables", "Load Template"]) -> (w430:string[])
      }
      frame "Check for RIO" {
        n333 = Unbundle By Name(w446) -> ("Desired System.Serial Number"=w440:string, "Desired System.ID"=w442:string, "Verification"=w444:bool, "StreamCtrlActive"=w443:bool)
        n334 = local read "RIO Found"() -> (w441:bool)
        n335 = case shown="False" w441 {
          selector: w441 -> [w452 _]
          tunnel: [string[] [] w460] -> w447
          tunnel: [w452 w459] -> w445
          tunnel: w444 -> [_ w458]
          tunnel: w443 -> [_ w457]
          tunnel: w442 -> [_ w456]
          tunnel: w440 -> [_ w453]
          frame True {
          }
          frame False {
            n336 = call "Find Network Systems.vi"() -> ("Serial Number"=w455:string)  [unwired: 10 in, 1 out]
            n337 = Equal?(x=w455, y=w453) -> (x = y?=w454:bool)
            n338 = case shown="True" w454 {
              selector: w454 -> [w463 w479]
              tunnel: w458 -> [w464 _]
              tunnel: [w465 string[] []] -> w460
              tunnel: [w463 w479] -> w459
              tunnel: w456 -> [w462 _]
              tunnel: w457 -> [w461 _]
              frame True {
                # "Desired system found."
                n339 = case shown="True" w461 {
                  tunnel: w462 -> [_ w466]
                  frame False {
                  }
                  frame True {
                    w467 = FALSE
                    n340 = Format Into String(format string="ni.var.psp://10.30.189.%s/Streaming Control/StreamCalibrated", w466) -> (resulting string=w473:string, error out=w474:errorcluster)  [unwired: 2 in]
                    n341 = shared-variable-open(w473, w474, w467) -> (w468:refnum<k21>, w471:errorcluster)  [unwired: 1 in]
                    n342 = shared-variable-write(w468, w471, w467) -> (w469:refnum<k21>, w470:errorcluster)
                    n343 = Close Variable Connection(8:w470, 11:w469) -> ()  [unwired: 1 out]
                  }
                }
                n344 = case shown="False" w464 {
                  tunnel: [string[] ["Load Targets", "Calculate Coeffs"] w476] -> w465
                  frame True {
                  }
                  frame False {
                    n345 = disable-structure shown="Enabled" {
                      disable-tunnel: [string[] ["Load Targets", "Start Cal"] string[] ["Load Targets"]] -> w476
                      frame Disabled {
                      }
                      frame Enabled {
                      }
                    }
                  }
                }
              }
              frame False {
                # "Couldn't find desired system."
                n346 = property on="Header" class="Bool"("DisabledEnum"=T10."Enabled" ("Disabled")) -> ()  [unwired: 2 in, 2 out]
                n347 = One Button Dialog(message="Couldn't connect to desired DAQ hardware.") -> ()  [unwired: 1 in, 1 out]
              }
            }
          }
        }
        "RIO Found" <- w445
        n348 = Insert Into Array(array=w449, index=0, new element=w447) -> (w448:string[])
      }
      frame "Adjust Channels" {
        w485 = T1[] [enum."V", enum."mA", enum."A", enum."Hz", enum."deg C"] items=["V", "mA", "A", "Hz", "deg C"]
        # "If the cal unit is disabled look for\nthe first non disabled cal unit"
        n349 = Unbundle By Name(w498) -> ("Cal Unit"=w493:T1, "Cal Target Array"=w488:string[], "Channel to Cal"=w484:T2)
        n350 = property on="Channel to Cal" class="Enum (strict)"() -> ("NumItems"=w490:u32)  [unwired: 2 in, 2 out]
        n351 = Index Array(array=w488, index=w484) -> (element=w487:string)
        n352 = for {
          N: w490 -> [_]
          shift-right: [w506] -> w489
          shift-left: i32[] [] ("Disabled Items []") -> [w507]
          i -> [w505]
          n353 = case shown="0..27, Default" w505 {
            tunnel: w507 -> [w508]
            tunnel: [w508] -> w506
            tunnel: w505 -> [_]
            frame 0..27, Default {
            }
          }
        }
        n354 = case shown="Default" w487 {
          tunnel: [0 ("index") 1 ("index") 2 ("index") 3 ("index") 4 ("index")] -> w486
          frame Default {
            # "9221\n9205"
          }
          frame "9208" {
            # "mA"
          }
          frame "A" {
          }
          frame "Hz" {
          }
          frame "9211" {
            # "degC"
          }
        }
        n355 = Delete From Array(array=w485, index=w486) -> (array with subset deleted=w483:T1[])  [unwired: 1 in, 1 out]
        n356 = Search 1D Array(1D array=w483, element=w493) -> (index of element=w495:i32)  [unwired: 1 in]
        n357 = Greater Or Equal To 0?(x=w495) -> (x >= 0?=w494:bool)
        n358 = property on="Channel to Cal" class="Enum (strict)"("Disabled Items []"=w489) -> ()  [unwired: 2 in, 2 out]
        n359 = property on="Cal Unit" class="Enum (strict)"("Disabled Items []"=w483) -> ()  [unwired: 2 in, 2 out]
        n360 = case shown="True" w494 {
          tunnel: [w509 w510] -> w492
          tunnel: w493 -> [w509 _]
          tunnel: w483 -> [_ w512]
          frame False {
          }
          frame True {
            n361 = for {
              N: 5 -> [_]
              tunnel: w512 -> [w516]
              tunnel: [w513] -> w510
              i -> [w513]
              stop <- w514 stop-if-true
              n362 = Search 1D Array(1D array=w516, element=w513) -> (index of element=w515:i32)  [unwired: 1 in]
              n363 = Less Than 0?(x=w515) -> (x < 0?=w514:bool)
            }
            n364 = local write "Cal Unit"(w510) -> ()
          }
        }
        n365 = Bundle By Name(cluster=w498, "Rack Version"=Rack_Version_Type_Def."cDAQ", "Cal Unit"=w492) -> (w497:T9)
      }
      frame "Clear Dev Data" {
        n366 = Bundle By Name(cluster=w519, "Verify Table"=string[][] [["", "", "", "", ""], ["", "", "", "", ""], ["", "", "", "", ""], ["", "", "", "", ""], ["", "", "", "", ""], ["", "", "", "", ""], ["", "", "", "", ""], ["", "", "", "", ""], ["", "", "", "", ""], ["", "", "", "", ""]]) -> (w518:T9)
      }
      frame "Update Dev Tables" {
        n367 = Unbundle By Name(w522) -> ("Verify Table"=w521:string[][])
        n368 = local write "Verify Table"(w521) -> ()
      }
      frame "Load Template" {
        n369 = Unbundle By Name(w525) -> ("Cal Template Path"=w530:path)
        n370 = call <vilib>:"Check if File or Folder Exists.vi"("path"=w530) -> ("file or folder exists?"=w529:bool)  [unwired: 8 in, 2 out]
        n371 = case shown="True" w529 {
          tunnel: [string[] [] string[] []] -> w528
          tunnel: w530 -> [w537 w540]
          tunnel: [FALSE ("Visible") FALSE ("Visible")] -> w531
          tunnel: [w534 w542] -> w532
          tunnel: [w534 w542] -> w533
          frame False {
            w534 = T10."Disabled and Grayed Out" ("Disabled")
            n372 = Format Into String(format string="Can't find cal spreadsheet template!\n\nShould have been here:  \"%s\"" ("message"), w537) -> (resulting string=w536:string)  [unwired: 2 in, 1 out]
            n373 = One Button Dialog(message=w536) -> ()  [unwired: 1 in, 1 out]
          }
          frame True {
            w542 = T10."Enabled" ("Disabled")
            n374 = call "Read Write Header.vi"("Cal Template Path"=w540, "Write (F)"=FALSE) -> ("Header Table 1"=w548:string[][], "Header Table 2"=w547:string[][], "Sys Cal Table"=w544:string[][], "Cal Standards Table"=w543:string[][], "Header Comments"=w545:string[][])  [unwired: 13 in]
            n375 = local write "Header Table 1"(w548) -> ()
            n376 = local write "Header Table 2"(w547) -> ()
            n377 = local write "Sys Cal Table"(w544) -> ()
            n378 = local write "Cal Standards Table"(w543) -> ()
            n379 = local write "Header Comments"(w545) -> ()
          }
        }
        n380 = property on="Load Indicator Tab" class="TabCtl (strict)"("Visible"=w531) -> ()  [unwired: 2 in, 2 out]
        n381 = property on="Header OK" class="Bool"("DisabledEnum"=w532) -> ()  [unwired: 2 in, 2 out]
        n382 = property on="Header Cancel" class="Bool"("DisabledEnum"=w533) -> ()  [unwired: 2 in, 2 out]
        n383 = Insert Into Array(array=w527, index=0, new element=w528) -> (w526:string[])
      }
      frame "Create Spreadsheet" {
        n384 = Unbundle By Name(w561) -> ("Rack Version"=w556:T8, "DAQ Rack"=w553:string, "Cal Files Base Path"=w563:path)
        n385 = Format Into String(format string="%s.xls", w553) -> (resulting string=w552:string)  [unwired: 2 in, 1 out]
        n386 = case shown="\"cDAQ\"" w556 {
          tunnel: ["DAQ Rack Cal Template.xls" ("name or relative path") "DAQ Cart Cal Template.xls" ("name or relative path") "New Durability Tank Cal Template.xls" ("name or relative path") "cDAQ Cal Template.xls" ("name or relative path")] -> w551
          frame Default {
          }
          frame "Cart" {
          }
          frame "RIO" {
          }
          frame "cDAQ" {
          }
        }
        n387 = Build Path(base path=w563, name or relative path=w552) -> (appended path=w550:path)
        n388 = Empty String/Path?(string/path=w553) -> (empty?=w555:bool)
        n389 = Not A Number/Path/Refnum?(number/path/refnum=w550) -> (NaN/Path/Refnum?=w565:bool)
        n390 = Or(x=w565, y=w555) -> (x .or. y?=w566:bool)
        n391 = Build Path(base path=w563, name or relative path=w551) -> (appended path=w564:path)
        n392 = case shown="True" w566 {
          tunnel: [string[] ["Save Header"] string[] []] -> w562
          tunnel: w550 -> [w572 _]
          tunnel: w564 -> [w573 _]
          frame False {
            n393 = call <vilib>:"Check if File or Folder Exists.vi"("path"=w572) -> ("file or folder exists?"=w571:bool)  [unwired: 8 in, 2 out]
            n394 = case shown="False" w571 {
              tunnel: w572 -> [w577 _]
              tunnel: w573 -> [w576 _]
              frame False {
                n395 = Copy(9:TRUE ("overwrite (F)"), 10:w577, 11:w576) -> ()  [unwired: 2 in, 3 out]
              }
              frame True {
              }
            }
          }
          frame True {
            w578 = T10."Enabled" ("Disabled")
            n396 = property on="Load Indicator Tab" class="TabCtl (strict)"("Visible"=FALSE) -> ()  [unwired: 2 in, 2 out]
            n397 = property on="Header OK" class="Bool"("DisabledEnum"=w578) -> ()  [unwired: 2 in, 2 out]
            n398 = property on="Header Cancel" class="Bool"("DisabledEnum"=w578) -> ()  [unwired: 2 in, 2 out]
            n399 = One Button Dialog(message="\"Manufacturer Serial #\" is blank or contains invalid characters.") -> ()  [unwired: 1 in, 1 out]
          }
        }
        n400 = Bundle By Name(cluster=w561, "Cal Spreadsheet Path"=w550) -> (w560:T9)
        n401 = Insert Into Array(array=w558, index=0, new element=w562) -> (w559:string[])
      }
      frame "Save Header" {
        n402 = Unbundle By Name(w590) -> ("Cal Spreadsheet Path"=w593:path, "Cal Template Path"=w594:path)
        n403 = Build Array(w593, w594) -> (w595:path[])
        n404 = for {
          tunnel: "Header Table 2" -> [w603]
          tunnel: "Sys Cal Table" -> [w602]
          tunnel: "Cal Standards Table" -> [w601]
          tunnel: "Header Comments" -> [w600]
          tunnel: [w599] -> w592
          tunnel: "Header Table 1" -> [w597]
          tunnel: w595 -> [w596] mode=indexing
          n405 = call "Read Write Header.vi"("Header Table 1 IN"=w597, "Header Table 2 IN"=w603, "Sys Cal Table IN"=w602, "Cal Standards Table IN"=w601, "Header Comments IN"=w600, "Cal Template Path"=w596, "Write (F)"=TRUE) -> ("Header Table 1"=w599:string[][])  [unwired: 8 in, 4 out]
        }
        n406 = flat-sequence {
          tunnel: w592 -> [_]
          frame #0 {
            w604 = T10."Enabled" ("Disabled")
            w606 = FALSE ("Visible")
            n407 = disable-structure shown="Disabled" {
              disable-tunnel: w604 -> [w607 _]
              frame Disabled {
                n408 = property on="Start Verification" class="Bool"("DisabledEnum"=w607) -> ()  [unwired: 2 in, 2 out]
              }
              frame Enabled {
              }
            }
            n409 = property on="View Spreadsheet" class="Bool"("DisabledEnum"=w604) -> ()  [unwired: 2 in, 2 out]
            n410 = property on="Main Tab" class="TabCtl (strict)"("DisabledEnum"=w604) -> ()  [unwired: 2 in, 2 out]
            n411 = property on="Tank IP:" class="Str"("DisabledEnum"=w604) -> ()  [unwired: 2 in, 2 out]
            n412 = property on="Channel to Cal" class="Enum (strict)"("DisabledEnum"=w604) -> ()  [unwired: 2 in, 2 out]
            n413 = property on="Start Cal" class="Bool"("DisabledEnum"=w604) -> ()  [unwired: 2 in, 2 out]
            n414 = property on="Cal Unit" class="Enum (strict)"("DisabledEnum"=T10."Enabled" ("Disabled")) -> ()  [unwired: 2 in, 2 out]
            n415 = property on="Load Indicator Tab" class="TabCtl (strict)"("Visible"=w606) -> ()  [unwired: 2 in, 2 out]
            n416 = property on="Header Tab" class="TabCtl (strict)"("Visible"=w606) -> ()  [unwired: 2 in, 2 out]
          }
        }
        n417 = Insert Into Array(array=w588, index=0, new element=string[] []) -> (w589:string[])
      }
      frame "Create Cal File" {
        n418 = Unbundle By Name(w611) -> ("Cal Files Base Path"=w613:path, "Cal Log Header"=w616:string[], "Default Cal Log"=w615:string[][])
        n419 = local read "Tank IP:"() -> (w608:string)
        n420 = Build Array (concatenate)(w616, w615) -> (w614:string[][])
        n421 = case shown="Default" w608 {
          tunnel: w614 -> [w625 _]
          tunnel: w613 -> [w624 _]
          tunnel: w608 -> [w622 _]
          tunnel: [w623 path "" ("dup path")] -> w609
          frame Default {
            n422 = Format Into String(format string="%s.cal", w622) -> (resulting string=w620:string)  [unwired: 2 in, 1 out]
            n423 = Build Path(base path=w624, name or relative path=w620) -> (appended path=w628:path)
            n424 = call <vilib>:"Check if File or Folder Exists.vi"("path"=w628) -> ("file or folder exists?"=w627:bool, "dup path"=w626:path)  [unwired: 8 in, 1 out]
            n425 = case shown="False" w627 {
              tunnel: w626 -> [w632 w633]
              tunnel: w625 -> [w631 _]
              tunnel: [w629 w633] -> w623
              frame False {
                n426 = call-poly <vilib>:"Write To Spreadsheet File.vi"("delimiter (\\t)"="," ("delimiter (\\t)"), "2D data"=w631, "file path (dialog if empty)"=w632) -> ("new file path (Not A Path if cancelled)"=w629:path)  [unwired: 5 in]
              }
              frame True {
              }
            }
          }
          frame "" {
          }
        }
        n427 = Bundle By Name(cluster=w611, "Cal File Path"=w609) -> (w610:T9)
        n428 = Insert Into Array(array=w617, index=0, new element=string[] ["Load Cal File"]) -> (w618:string[])
      }
      frame "Load Cal File" {
        n429 = Unbundle By Name(w639) -> ("Default Cal Log"=w635:string[][], "Cal File Path"=w636:path)
        n430 = Empty String/Path?(string/path=w636) -> (empty?=w637:bool)
        n431 = case shown="False" w637 {
          tunnel: w636 -> [w646 _]
          tunnel: [w650 w680] -> w643
          tunnel: [w648 string[] []] -> w640
          tunnel: w639 -> [w647 w680]
          tunnel: w635 -> [w644 _]
          frame False {
            n432 = call <vilib>:"Check if File or Folder Exists.vi"("path"=w646) -> ("file or folder exists?"=w649:bool, "dup path"=w645:path)  [unwired: 8 in, 1 out]
            n433 = case shown="True" w649 {
              tunnel: w645 -> [_ w673]
              tunnel: w647 -> [w651 w670]
              tunnel: [w651 w669] -> w650
              tunnel: [string[] ["Create Cal File"] string[] []] -> w648
              tunnel: w644 -> [_ w666]
              frame False {
              }
              frame True {
                w665 = 0 ("index (row)")
                n434 = call-poly <vilib>:"Read From Spreadsheet File.vi"("delimiter (\\t)"="," ("delimiter (\\t)"), "file path (dialog if empty)"=w673) -> ("all rows"=w672:string[][])  [unwired: 5 in, 4 out]
                n435 = Delete From Array(array=w672, index (row)=0) -> (array with subset deleted=w661:string[][])  [unwired: 2 in, 1 out]
                n436 = Index Array(array=w661, index (col)=0 ("disabled index (col)")) -> (element=w663:string[])  [unwired: 1 in]
                n437 = Search 1D Array(1D array=w663, element="") -> (index of element=w659:i32)  [unwired: 1 in]
                n438 = Delete From Array(array=w661, index (row)=w659) -> (array with subset deleted=w660:string[][])  [unwired: 2 in, 1 out]
                n439 = Replace Array Subset(array=w666, new element=w660, index (row)=w665, index (col)=w665) -> (w657:string[][])
                n440 = Index Array(array=w657, index (col)=1 ("disabled index (col)")) -> (element=w654:string[])  [unwired: 1 in]
                n441 = for {
                  tunnel: w654 -> [w675] mode=indexing
                  tunnel: [w674] -> w653 mode=indexing
                  n442 = case shown="\"9211\"" w675 {
                    tunnel: ["V" "mA" "degC"] -> w674
                    frame Default {
                    }
                    frame "9208" {
                    }
                    frame "9211" {
                    }
                  }
                }
                n443 = Replace Array Subset(array=w657, new element=w653, index (col)=1 ("disabled index (col)")) -> (w656:string[][])  [unwired: 1 in]
                n444 = Bundle By Name(cluster=w670, "Cal Log"=w656) -> (w669:T9)
                n445 = property on="Cal Table" class="Tbl (strict)"("Value"=w656) -> ()  [unwired: 2 in, 2 out]
              }
            }
          }
          frame True {
          }
        }
        n446 = Insert Into Array(array=w641, index=0, new element=w640) -> (w642:string[])
      }
      frame "Load Targets" {
        w737 = 0 ("length")
        # "#Change In \"A\" selection added selection of \"RIO\" that links 25A Targets and Setpoints"
        n447 = Unbundle By Name(w740) -> ("Cal Log"=w705:string[][], "Cal Targets Path"=w747:path, "cDAQ Targets"=w742:T3, "Cal Target Array"=w727:string[], "Verify Table"=w694:string[][], "Channel to Cal"=w716:T2)
        n448 = property on="Cancel Verify" class="Bool"("DisabledEnum"=T10."Enabled" ("Disabled")) -> ()  [unwired: 2 in, 2 out]
        n449 = property on="Cal Table" class="Tbl (strict)"("Active Cell"=T12 {"Row"=-2, "Column"=-2} ("Active Cell:Active Cell"), "Cell BG Color"=u32 16448250) -> ()  [unwired: 2 in, 2 out]
        n450 = Index Array(array=w705, index (row)=w716) -> (element=w726:string[])  [unwired: 1 in]
        n451 = call <vilib>:"Open Config Data.vi"("configuration file path"=w747) -> ("error out"=w745:errorcluster, "refnum"=w746:T15)  [unwired: 8 in, 1 out]
        n452 = Array Subset "Calibration"(array=w726, index=2, length=10) -> (w689:string[])
        n453 = Array Subset "Verification"(array=w726, index=18, length=20) -> (w696:string[])
        n454 = property on="Apply Cal" class="Bool"("DisabledEnum"=T10."Disabled and Grayed Out" ("Disabled")) -> ()  [unwired: 2 in, 2 out]
        n455 = call <userlib>:"Read INI Cluster__ogtk.vi"("error in (no error)"=w745, "INI Fomatted Cluster Type"=w742, "refnum"=w746) -> ("error out"=w743:errorcluster, "INI Fomatted Cluster"=w741:variant, "dup refnum"=w744:T15)  [unwired: 4 in, 2 out]
        n456 = Index Array(array=w696, index #1=1 ("index"), index #2=3 ("index"), index #3=5 ("index"), index #4=7 ("index"), index #5=9 ("index")) -> (element #1=w715:string, element #2=w712:string, element #3=w714:string, element #4=w711:string, element #5=w713:string)
        n457 = call <vilib>:"Close Config Data.vi"("error in (no error)"=w743, "refnum"=w744) -> ()  [unwired: 8 in, 2 out]
        n458 = Fract/Exp String To Number(string=w689) -> (number=w699:dbl[])  [unwired: 3 in, 1 out]
        n459 = Empty Array?(array=w689) -> ()  [unwired: 1 out]
        n460 = Empty String/Path?(string/path=w715) -> (empty?=w708:bool)
        n461 = Empty String/Path?(string/path=w714) -> (empty?=w707:bool)
        n462 = Empty String/Path?(string/path=w713) -> (empty?=w706:bool)
        n463 = Variant To Data(type=w742, Variant=w741) -> (data=w730:T3)  [unwired: 1 in, 1 out]
        n464 = Index Array(array=w727, index=w716) -> (element=w731:string)
        n465 = Empty String/Path?(string/path=w712) -> (empty?=w710:bool)
        n466 = Empty String/Path?(string/path=w711) -> (empty?=w709:bool)
        n467 = Compound Arithmetic op=AND(w708, w710, w707, w709, w706) -> (w690:bool)
        n468 = case shown="\"9211\"" w731 {
          tunnel: w730 -> [w795 w798 w801 w804]
          tunnel: [w793 w796 w799 w802] -> w728
          tunnel: [w794 w797 w800 w803] -> w729
          frame "9221", Default {
            n469 = Unbundle By Name(w795) -> ("9221 Targets"=w794:T4, "9221 Setpoints"=w793:T5)
          }
          frame "9205" {
            n470 = Unbundle By Name(w798) -> ("9205 Targets"=w797:T4, "9205 Setpoints"=w796:T5)
          }
          frame "9208" {
            n471 = Unbundle By Name(w801) -> ("9208 Targets"=w800:T4, "9208 Setpoints"=w799:T5)
          }
          frame "9211" {
            n472 = Unbundle By Name(w804) -> ("9211 Targets"=w803:T4, "9211 Setpoints"=w802:T5)
          }
        }
        n473 = case shown="True" w690 {
          tunnel: w696 -> [_ w768]
          tunnel: w694 -> [w760 w767]
          tunnel: [w760 w761] -> w693
          frame True {
          }
          frame False {
            n474 = for {
              tunnel: w768 -> [w774] mode=indexing
              tunnel: [w774] -> w763 mode=indexing if=w770
              tunnel: [w774] -> w762 mode=indexing if=w769
              i -> [w773]
              n475 = Quotient & Remainder(x=w773, y=2) -> (x-y*floor(x/y)=w771:i32)  [unwired: 1 out]
              n476 = Equal To 0?(x=w771) -> (x = 0?=w770:bool)
              n477 = Not(x=w770) -> (.not. x?=w769:bool)
            }
            n478 = Replace Array Subset(array=w767, new element=w763, index (col)=0 ("disabled index (col)")) -> (w766:string[][])  [unwired: 1 in]
            n479 = Replace Array Subset(array=w766, new element=w762, index (col)=1 ("disabled index (col)")) -> (w761:string[][])  [unwired: 1 in]
          }
        }
        n480 = case shown="False" w690 {
          tunnel: w692 -> [w757 w759]
          tunnel: [w756 w759] -> w691
          frame False {
            n481 = Insert Into Array(array=w757, index=0, new element=string[] ["Calc Dev"]) -> (w756:string[])
          }
          frame True {
          }
        }
        n482 = for {
          tunnel: w689 -> [w754] mode=indexing
          tunnel: [w753] -> w688 mode=indexing
          n483 = Empty String/Path?(string/path=w754) -> (empty?=w753:bool)
        }
        n484 = Cluster To Array(cluster=w729) -> (array=w738:dbl[])
        n485 = Cluster To Array(cluster=w728) -> (array=w695:dbl[])
        n486 = And Array Elements(Boolean array=w688) -> (logical AND=w687:bool)
        n487 = Delete From Array(array=w738, length=w737, index=w737) -> (deleted portion=w733:dbl[], array with subset deleted=w736:dbl[])
        n488 = call-poly <userlib>:"Remove Duplicates from 1D Array__ogtk.vi"("Input Array"=w736) -> ("Output Array"=w735:dbl[])  [unwired: 1 out]
        n489 = Build Array (concatenate)(w733, w735) -> (w734:dbl[])
        n490 = Number To Fractional String(number=w734, precision (6)=i16 3) -> (F-format string=w739:string[])  [unwired: 2 in]
        n491 = case shown="False" w687 {
          tunnel: w695 -> [_ w792]
          tunnel: [w780 w791] -> w704
          tunnel: [w784 w790] -> w703
          tunnel: [w783 w789] -> w702
          tunnel: [w782 w788] -> w701
          tunnel: [w781 w787] -> w700
          tunnel: w699 -> [w785 _]
          tunnel: [w779 w786] -> w686
          tunnel: [w778 w786] -> w685
          tunnel: [w777 w786] -> w684
          tunnel: [w776 w786] -> w683
          tunnel: [w775 w786] -> w682
          frame False {
            n492 = Index Array(array=w785) -> (element #1=w779:dbl, element #2=w784:dbl, element #3=w778:dbl, element #4=w783:dbl, element #5=w777:dbl, element #6=w782:dbl, element #7=w776:dbl, element #8=w781:dbl, element #9=w775:dbl, element #10=w780:dbl)  [unwired: 10 in]
          }
          frame True {
            w786 = 0.0 ("Label")
            n493 = Index Array(array=w792) -> (element #1=w790:dbl, element #2=w789:dbl, element #3=w788:dbl, element #4=w787:dbl, element #5=w791:dbl)  [unwired: 5 in]
          }
        }
        n494 = Replace Array Subset(array=w694, new element=w739, index (col)=0 ("disabled index (col)")) -> (w698:string[][])  [unwired: 1 in]
        n495 = Select(t=w698, s=w690, f=w693) -> (s? t:f=w697:string[][])
        n496 = local write "Reading Value 1"(w686) -> ()
        n497 = local write "Reading Value 2"(w685) -> ()
        n498 = local write "Reading Value 3"(w684) -> ()
        n499 = local write "Reading Value 4"(w683) -> ()
        n500 = local write "Reading Value 5"(w682) -> ()
        n501 = local write "Cal Value 1"(w703) -> ()
        n502 = local write "Cal Value 2"(w702) -> ()
        n503 = local write "Cal Value 3"(w701) -> ()
        n504 = local write "Cal Value 4"(w700) -> ()
        n505 = local write "Cal Value 5"(w704) -> ()
        n506 = Bundle By Name(cluster=w740, "cDAQ Targets"=w730, "Verify Table"=w697) -> (w749:T9)
        n507 = property on="Verify Table" class="Tbl (strict)"("Value"=w697) -> ()  [unwired: 2 in, 2 out]
      }
      frame "Start Cal" {
        w805 = T10."Disabled and Grayed Out" ("Disabled")
        w808 = T10."Enabled" ("Disabled")
        n508 = property on="Header" class="Bool"("DisabledEnum"=w805) -> ()  [unwired: 2 in, 2 out]
        n509 = property on="Channel to Cal" class="Enum (strict)"("DisabledEnum"=w805) -> ()  [unwired: 2 in, 2 out]
        n510 = property on="View Spreadsheet" class="Bool"("DisabledEnum"=w805) -> ()  [unwired: 2 in, 2 out]
        n511 = property on="Cal Tab" class="TabCtl (strict)"("Visible"=TRUE) -> ()  [unwired: 2 in, 2 out]
        n512 = property on="Start Cal" class="Bool"("DisabledEnum"=w805) -> ()  [unwired: 2 in, 2 out]
        n513 = disable-structure shown="Disabled" {
          disable-tunnel: w805 -> [w810 _]
          frame Disabled {
            n514 = property on="Cal Unit" class="Enum (strict)"("DisabledEnum"=w810) -> ()  [unwired: 2 in, 2 out]
          }
          frame Enabled {
          }
        }
        n515 = property on="Start Verification" class="Bool"("DisabledEnum"=w805) -> ()  [unwired: 2 in, 2 out]
        n516 = property on="Reading Value 1" class="DigNum (strict)"("DisabledEnum"=w808) -> ()  [unwired: 2 in, 2 out]
        n517 = property on="Cal Value 1" class="DigNum (strict)"("DisabledEnum"=w808) -> ()  [unwired: 2 in, 2 out]
        n518 = property on="1st Point Cal" class="Bool (strict)"("DisabledEnum"=w808) -> ()  [unwired: 2 in, 2 out]
        n519 = property on="Reading Value 2" class="DigNum (strict)"("DisabledEnum"=w808) -> ()  [unwired: 2 in, 2 out]
        n520 = property on="Cal Value 2" class="DigNum (strict)"("DisabledEnum"=w808) -> ()  [unwired: 2 in, 2 out]
        n521 = property on="2nd Point Cal" class="Bool (strict)"("DisabledEnum"=w808) -> ()  [unwired: 2 in, 2 out]
        n522 = property on="Reading Value 3" class="DigNum (strict)"("DisabledEnum"=w808) -> ()  [unwired: 2 in, 2 out]
        n523 = property on="Cal Value 3" class="DigNum (strict)"("DisabledEnum"=w808) -> ()  [unwired: 2 in, 2 out]
        n524 = property on="3rd Point Cal" class="Bool (strict)"("DisabledEnum"=w808) -> ()  [unwired: 2 in, 2 out]
        n525 = property on="Reading Value 4" class="DigNum (strict)"("DisabledEnum"=w808) -> ()  [unwired: 2 in, 2 out]
        n526 = property on="Cal Value 4" class="DigNum (strict)"("DisabledEnum"=w808) -> ()  [unwired: 2 in, 2 out]
        n527 = property on="4th Point Cal" class="Bool (strict)"("DisabledEnum"=w808) -> ()  [unwired: 2 in, 2 out]
        n528 = property on="Reading Value 5" class="DigNum (strict)"("DisabledEnum"=w808) -> ()  [unwired: 2 in, 2 out]
        n529 = property on="Cal Value 5" class="DigNum (strict)"("DisabledEnum"=w808) -> ()  [unwired: 2 in, 2 out]
        n530 = property on="5th Point Cal" class="Bool (strict)"("DisabledEnum"=w808) -> ()  [unwired: 2 in, 2 out]
      }
      frame "Calibrating 1".."Calibrating 6" {
        # "When it said \"Calibrating 1\"..\"Calibrating 5\" it was not accepting Calibrating 5"
        n531 = case shown="\"Calibrating 4\"" w816 {
          tunnel: [0.0 w822 w824 w826 w828 w830] -> w815
          tunnel: [1 1 2 3 4 5] -> w811
          frame Default {
          }
          frame "Calibrating 1" {
            n532 = local read "Cal Value 1"() -> (w822:dbl)
          }
          frame "Calibrating 2" {
            n533 = local read "Cal Value 2"() -> (w824:dbl)
          }
          frame "Calibrating 3" {
            n534 = local read "Cal Value 3"() -> (w826:dbl)
          }
          frame "Calibrating 4" {
            n535 = local read "Cal Value 4"() -> (w828:dbl)
          }
          frame "Calibrating 5" {
            n536 = local read "Cal Value 5"() -> (w830:dbl)
          }
        }
        n537 = property on="Cal Tab" class="TabCtl (strict)"("Visible"=TRUE) -> ()  [unwired: 2 in, 2 out]
        n538 = local write "Cal Tab"(enum32{"Apply", "Cal"}."Cal" ("Cal Tab")) -> ()
        n539 = local write "Master Value"(w815) -> ()
        n540 = Bundle By Name(cluster=w813, "LastCalPt"=w811) -> (w812:T9)
      }
      frame "Stop Calibrating" {
        n541 = local write "Cal Tab"(enum32{"Apply", "Cal"}."Apply" ("Cal Tab")) -> ()
      }
      frame "Calculate Coeffs" {
        w835 = T10."Enabled" ("Disabled")
        # "Used to enable and start the verification from here"
        n542 = Unbundle By Name(w842) -> ("Channel to Cal"=w838:T2, "Cal Unit"=w841:T1, "Verification"=w840:bool, "Cal Log"=w839:string[][])
        n543 = case shown="False" w840 {
          tunnel: [w856 w883] -> w847
          tunnel: [w855 w882] -> w846
          tunnel: [w854 w881] -> w845
          tunnel: w841 -> [w853 w880]
          tunnel: w839 -> [_ w884]
          tunnel: w838 -> [_ w885]
          tunnel: [w852 w879] -> w837
          tunnel: [w851 w878] -> w836
          frame False {
            n544 = case shown="\"deg C\"" w853 {
              tunnel: [w873 w876] -> w856
              tunnel: [w872 1.0] -> w855
              tunnel: [w871 w876] -> w854
              tunnel: [w866 w876] -> w852
              tunnel: [w865 w876] -> w851
              frame "V", "Hz", Default {
                n545 = local read "Reading Value 1"() -> (w864:dbl)
                n546 = local read "Reading Value 2"() -> (w863:dbl)
                n547 = local read "Reading Value 3"() -> (w862:dbl)
                n548 = local read "Reading Value 4"() -> (w860:dbl)
                n549 = local read "Reading Value 5"() -> (w859:dbl)
                n550 = Build Array("Cal Value 1", "Cal Value 2", "Cal Value 3", "Cal Value 4", "Cal Value 5") -> (w870:dbl[])
                n551 = Build Array(w864, w863, w862, w860, w859) -> (w869:dbl[])
                n552 = call <vilib>:"General Polynomial Fit Coefficients.vi"("Y"=w870, "polynomial order"=4, "X"=w869) -> ("Polynomial Coefficients"=w868:dbl[])  [unwired: 11 in, 1 out]
                n553 = Index Array(array=w868) -> (element #1=w873:dbl, element #2=w872:dbl, element #3=w871:dbl, element #4=w866:dbl, element #5=w865:dbl)  [unwired: 5 in]
              }
              frame "deg C" {
                w876 = 0.0
              }
            }
          }
          frame True {
            n554 = case shown="Default" w880 {
              selector: w880 -> [w888 _]
              tunnel: w885 -> [w904 _]
              tunnel: w884 -> [w896 _]
              tunnel: [w891 w910] -> w883
              tunnel: [w890 1.0 ("Label")] -> w882
              tunnel: [w889 w910] -> w881
              tunnel: [w887 w910] -> w879
              tunnel: [w886 w910] -> w878
              frame Default {
                n555 = Format Into String(w904) -> (resulting string=w901:string)  [unwired: 3 in, 1 out]
                n556 = Format Into String(w888) -> (resulting string=w897:string)  [unwired: 3 in, 1 out]
                n557 = Index Array(array=w896, index (col) #1=0 ("disabled index (col)"), index (col) #2=1 ("index (col)")) -> (element #1=w902:string[], element #2=w898:string[])  [unwired: 2 in]
                n558 = call-poly <userlib>:"Search Array__ogtk.vi"("Array"=w902, "Element Data"=w901) -> ("Indices of Elements"=w899:i32[])  [unwired: 7 in]
                n559 = for {
                  tunnel: w899 -> [w905] mode=indexing
                  tunnel: w898 -> [w909]
                  tunnel: w897 -> [w907]
                  tunnel: [w905] -> w895
                  stop <- w906 stop-if-true
                  n560 = Index Array(array=w909, index=w905) -> (element=w908:string)
                  n561 = Equal?(x=w907, y=w908) -> (x = y?=w906:bool)
                }
                n562 = Index Array(array=w896, index (row)=w895) -> (element=w894:string[])  [unwired: 1 in]
                n563 = Fract/Exp String To Number(string=w894) -> (number=w893:dbl[])  [unwired: 3 in, 1 out]
                n564 = Index Array(array=w893, index #1=12 ("index")) -> (element #1=w891:dbl, element #2=w890:dbl, element #3=w889:dbl, element #4=w887:dbl, element #5=w886:dbl)  [unwired: 4 in]
              }
              frame "deg C" {
                w910 = 0.0 ("Label")
              }
            }
          }
        }
        "a0" <- w847
        "a2" <- w845
        "a1" <- w846
        "a4" <- w836
        "a3" <- w837
        n565 = property on="Cal Table" class="Tbl (strict)"("DisabledEnum"=T10."Disabled and Grayed Out" ("Disabled")) -> ()  [unwired: 2 in, 2 out]
        n566 = property on="Save Cal" class="Bool"("DisabledEnum"=T10."Enabled" ("Disabled")) -> ()  [unwired: 2 in, 2 out]
        n567 = Insert Into Array(array=w848, index=0, new element=string[] ["Save Calibration"]) -> (w849:string[])
        n568 = property on="a0" class="DigNum (strict)"("DisabledEnum"=w835) -> ()  [unwired: 2 in, 2 out]
        n569 = property on="a1" class="DigNum (strict)"("DisabledEnum"=w835) -> ()  [unwired: 2 in, 2 out]
        n570 = property on="a2" class="DigNum (strict)"("DisabledEnum"=w835) -> ()  [unwired: 2 in, 2 out]
        n571 = property on="a3" class="DigNum (strict)"("DisabledEnum"=w835) -> ()  [unwired: 2 in, 2 out]
        n572 = property on="a4" class="DigNum (strict)"("DisabledEnum"=w835) -> ()  [unwired: 2 in, 2 out]
      }
      frame "Cal Review Prep" {
        w917 = T10."Disabled and Grayed Out" ("Disabled")
        n573 = Unbundle By Name(w918) -> ("Desired System.ID"=w919:string)
        n574 = Format Into String(format string="ni.var.psp://10.30.189.%s/Streaming Control/StreamCalibrated", w919) -> (resulting string=w927:string, error out=w928:errorcluster)  [unwired: 2 in]
        n575 = property on="Cal Tab" class="TabCtl (strict)"("Visible"=FALSE) -> ()  [unwired: 2 in, 2 out]
        n576 = property on="Verify Tab" class="TabCtl (strict)"("Visible"=TRUE) -> (error out=w914:errorcluster)  [unwired: 2 in, 1 out]
        n577 = shared-variable-open(w927, w928, FALSE) -> (w921:refnum<k21>, w924:errorcluster)  [unwired: 1 in]
        n578 = shared-variable-write(w921, w924, TRUE ("data in")) -> (w922:refnum<k21>, w923:errorcluster)
        n579 = property on="Verify Table" class="Tbl (strict)"(error in=w914, "Key Focus"=TRUE, "EditPos"=T12 {"Row"=0, "Column"=1} ("Active Cell:Active Cell")) -> ()  [unwired: 1 in, 2 out]
        n580 = Close Variable Connection(8:w923, 11:w922) -> ()  [unwired: 1 out]
        n581 = Insert Into Array(array=w932, index=0, new element=string[] ["Cal Review"]) -> (w931:string[])
        n582 = property on="Reading Value 1" class="DigNum (strict)"("DisabledEnum"=w917) -> ()  [unwired: 2 in, 2 out]
        n583 = property on="Cal Value 1" class="DigNum (strict)"("DisabledEnum"=w917) -> ()  [unwired: 2 in, 2 out]
        n584 = property on="1st Point Cal" class="Bool (strict)"("DisabledEnum"=w917) -> ()  [unwired: 2 in, 2 out]
        n585 = property on="Reading Value 2" class="DigNum (strict)"("DisabledEnum"=w917) -> ()  [unwired: 2 in, 2 out]
        n586 = property on="Cal Value 2" class="DigNum (strict)"("DisabledEnum"=w917) -> ()  [unwired: 2 in, 2 out]
        n587 = property on="2nd Point Cal" class="Bool (strict)"("DisabledEnum"=w917) -> ()  [unwired: 2 in, 2 out]
        n588 = property on="Reading Value 3" class="DigNum (strict)"("DisabledEnum"=w917) -> ()  [unwired: 2 in, 2 out]
        n589 = property on="Cal Value 3" class="DigNum (strict)"("DisabledEnum"=w917) -> ()  [unwired: 2 in, 2 out]
        n590 = property on="3rd Point Cal" class="Bool (strict)"("DisabledEnum"=w917) -> ()  [unwired: 2 in, 2 out]
        n591 = property on="Reading Value 4" class="DigNum (strict)"("DisabledEnum"=w917) -> ()  [unwired: 2 in, 2 out]
        n592 = property on="Cal Value 4" class="DigNum (strict)"("DisabledEnum"=w917) -> ()  [unwired: 2 in, 2 out]
        n593 = property on="4th Point Cal" class="Bool (strict)"("DisabledEnum"=w917) -> ()  [unwired: 2 in, 2 out]
        n594 = property on="Reading Value 5" class="DigNum (strict)"("DisabledEnum"=w917) -> ()  [unwired: 2 in, 2 out]
        n595 = property on="Cal Value 5" class="DigNum (strict)"("DisabledEnum"=w917) -> ()  [unwired: 2 in, 2 out]
        n596 = property on="5th Point Cal" class="Bool (strict)"("DisabledEnum"=w917) -> ()  [unwired: 2 in, 2 out]
      }
      frame "Cal Review" {
        n597 = Unbundle By Name(w943) -> ("Auto"=w941:bool, "Verify Table"=w944:string[][])
        n598 = property on="Verify Table" class="Tbl (strict)"() -> ("EditPos"=w957:T12)  [unwired: 2 in, 2 out]
        n599 = Unbundle(w957) -> ("Row"=w955:i32)  [unwired: 1 out]
        n600 = local read "Ver Reading"() -> (w934:dbl)
        n601 = Greater Or Equal To 0?(x=w955) -> (x >= 0?=w956:bool)
        n602 = Index Array(array=w944, index (row)=w955, index (col)=0 ("disabled index (col)")) -> (element=w947:string)
        n603 = Fract/Exp String To Number(string=w947) -> (number=w936:dbl)  [unwired: 3 in, 1 out]
        n604 = case shown="True" w956 {
          tunnel: w955 -> [_ w965]
          frame False {
          }
          frame True {
            "Row" <- w965
          }
        }
        n605 = Increment(x=w934) -> (x+1=w948:dbl)
        n606 = Increment(x=w936) -> (x+1=w949:dbl)
        n607 = Subtract(x=w948, y=w949) -> (x-y=w937:dbl)
        n608 = Divide(x=w937, y=w948) -> (x/y=w953:dbl)
        n609 = local read "Lost Connection"() -> (w933:bool)
        n610 = Empty String/Path?(string/path=w947) -> (empty?=w940:bool)
        n611 = Absolute Value(x=w953) -> (abs(x)=w935:dbl)
        n612 = Not(x=w940) -> (.not. x?=w950:bool)
        n613 = Less?(x=w935, y=0.1) -> (x < y?=w951:bool)
        n614 = Compound Arithmetic op=AND(w941, w951, w950) -> (w946:bool)
        n615 = call "Reading Delay.vi"("Delay"="ms", "In Range"=w946) -> ("Take Reading"=w939:bool)  [unwired: 9 in]
        n616 = case shown="False" w933 {
          tunnel: [string[] ["Main", "Cal Review"] string[] ["End Cal"]] -> w961
          frame False {
          }
          frame True {
          }
        }
        n617 = case shown="True" w939 {
          selector: w939 -> [_ w964]
          frame False {
          }
          frame True {
            n618 = property on="Verify Read" class="Bool (strict)"("Val(Sgnl)"=w964) -> ()  [unwired: 2 in, 2 out]
          }
        }
        n619 = Bundle By Name(cluster=w943, "Init Mean"=FALSE) -> (w938:T9)
        n620 = Insert Into Array(array=w959, index=0, new element=w961) -> (w960:string[])
      }
      frame "Stop Verification" {
        w966 = T10."Enabled" ("Disabled")
        n621 = property on="Header" class="Bool"("DisabledEnum"=w966) -> ()  [unwired: 2 in, 2 out]
        n622 = property on="Channel to Cal" class="Enum (strict)"("DisabledEnum"=w966) -> ()  [unwired: 2 in, 2 out]
        n623 = property on="View Spreadsheet" class="Bool"("DisabledEnum"=w966) -> ()  [unwired: 2 in, 2 out]
        n624 = property on="Cal Unit" class="Enum (strict)"("DisabledEnum"=T10."Enabled" ("Disabled")) -> ()  [unwired: 2 in, 2 out]
        n625 = property on="Start Cal" class="Bool"("DisabledEnum"=w966) -> ()  [unwired: 2 in, 2 out]
        n626 = disable-structure shown="Disabled" {
          disable-tunnel: w966 -> [w971 _]
          frame Disabled {
            n627 = property on="Start Verification" class="Bool"("DisabledEnum"=w971) -> ()  [unwired: 2 in, 2 out]
          }
          frame Enabled {
          }
        }
        n628 = property on="Verify Tab" class="TabCtl (strict)"("Visible"=FALSE) -> ()  [unwired: 2 in, 2 out]
      }
      frame "Save Cal" {
        w1018 = u16 4 ("y")
        n629 = Unbundle By Name(w993) -> ("Cal File Path"=w1003:path, "Cal Log Header"=w1025:string[], "Cal Log"=w989:string[][], "Channel to Cal"=w1001:T2, "Cal Unit"=w1002:T1, "Verification"=w992:bool, "Verify Table"=w1004:string[][])
        n630 = local read "Reading Value 1"() -> (w986:dbl)
        n631 = local read "Reading Value 2"() -> (w984:dbl)
        n632 = local read "Reading Value 3"() -> (w982:dbl)
        n633 = local read "Reading Value 4"() -> (w980:dbl)
        n634 = local read "Reading Value 5"() -> (w978:dbl)
        n635 = local read "Cal Value 1"() -> (w985:dbl)
        n636 = local read "Cal Value 2"() -> (w983:dbl)
        n637 = local read "Cal Value 3"() -> (w981:dbl)
        n638 = local read "Cal Value 4"() -> (w979:dbl)
        n639 = local read "Cal Value 5"() -> (w977:dbl)
        n640 = local read "a0"() -> (w976:dbl)
        n641 = local read "a1"() -> (w975:dbl)
        n642 = local read "a2"() -> (w974:dbl)
        n643 = local read "a3"() -> (w973:dbl)
        n644 = local read "a4"() -> (w972:dbl)
        n645 = Build Array(w986, w985, w984, w983, w982, w981, w980, w979, w978, w977, w976, w975, w974, w973, w972) -> (w1031:dbl[])
        n646 = Format Into String(w1001) -> (resulting string=w997:string)  [unwired: 3 in, 1 out]
        n647 = Format Into String(w1002) -> (resulting string=w994:string)  [unwired: 3 in, 1 out]
        n648 = Index Array(array=w989, index (col) #1=0 ("disabled index (col)"), index (col) #2=1 ("index (col)")) -> (element #1=w998:string[], element #2=w996:string[])  [unwired: 2 in]
        n649 = Search 1D Array(1D array=w998, element=w997) -> (index of element=w995:i32)  [unwired: 1 in]
        n650 = disable-structure shown="Enabled" {
          disable-tunnel: w996 -> [w1038 _]
          disable-tunnel: w995 -> [w1037 w1039]
          disable-tunnel: w994 -> [w1036 _]
          disable-tunnel: [w1035 w1039] -> w988
          frame Disabled {
            n651 = Search 1D Array(1D array=w1038, element=w1036, start index (0)=w1037) -> (index of element=w1035:i32)
          }
          frame Enabled {
          }
        }
        n652 = Index Array(array=w1004, index (col) #1=0 ("disabled index (col)"), index (col) #2=1 ("disabled index (col)")) -> (element #1=w1008:string[], element #2=w1007:string[])  [unwired: 2 in]
        n653 = Format Date/Time String(time format string (%c)="%d%b%y %I:%M:%S %p") -> (date/time string=w1029:string)  [unwired: 2 in]
        n654 = Interleave 1D Arrays(w1008, w1007) -> (w1006:string[])
        n655 = Index Array(array=w989, index (row)=w988) -> (element=w987:string[])  [unwired: 1 in]
        n656 = To Upper Case(1:w1029) -> (0:w991:string)
        n657 = case shown="True" w992 {
          tunnel: w1031 -> [w1043 _]
          tunnel: [w1041 w1045] -> w1030
          tunnel: [w1040 w1044] -> w990
          tunnel: w991 -> [w1040 _]
          tunnel: w987 -> [_ w1047]
          frame False {
            n658 = Number To Fractional String(number=w1043, precision (6)=i16 16) -> (F-format string=w1041:string[])  [unwired: 2 in]
          }
          frame True {
            n659 = Array Subset(array=w1047, index=2, length=9) -> (w1045:string[])
            n660 = Index Array(array=w1047, index=11) -> (element=w1044:string)
          }
        }
        n661 = Build Array (concatenate)(w997, w994, w1030, w990, w1006) -> (w1027:string[])
        n662 = Greater?(x=w988, y=w1018) -> (0:w1017:bool)
        n663 = Subtract(x=w988, y=w1018) -> (x-y=w1016:i32)
        n664 = Bundle(cluster=T12 {"Row"=0, "Column"=0} ("Active Cell:Active Cell"), "Row"=w988, "Column"=-2) -> (w1019:T12)
        n665 = Select(t=w1016, s=w1017, f=u16 0 ("y")) -> (s? t:f=w1013:i32)
        n666 = Replace Array Subset(array=w989, new element=w1027, index (row)=w988) -> (w1024:string[][])  [unwired: 1 in]
        n667 = Bundle(cluster=T12 {"Row"=0, "Column"=0} ("Active Cell:Active Cell"), "Row"=w1013, "Column"=0) -> (w1012:T12)
        n668 = Build Array (concatenate)(w1025, w1024) -> (w1023:string[][])
        n669 = Insert Into Array(array=w1032, index=0, new element=string[] ["Write to Excel", "Load Cal File", "End Cal", "Increment Channel"]) -> (w1033:string[])
        n670 = property on="Cal Table" class="Tbl (strict)"("Active Cell"=w1019, "Cell BG Color"=u32 16775793, "Index Values"=w1012) -> ()  [unwired: 2 in, 2 out]
        n671 = call-poly <vilib>:"Write To Spreadsheet File.vi"("delimiter (\\t)"="," ("delimiter (\\t)"), "2D data"=w1023, "file path (dialog if empty)"=w1003) -> ()  [unwired: 5 in, 1 out]
      }
      frame "Save Calibration" {
        w1096 = u16 4 ("y")
        n672 = Unbundle By Name(w1071) -> ("Cal File Path"=w1081:path, "Cal Log Header"=w1103:string[], "Cal Log"=w1067:string[][], "Channel to Cal"=w1079:T2, "Cal Unit"=w1080:T1, "Verification"=w1070:bool, "Verify Table"=w1082:string[][])
        n673 = local read "Reading Value 1"() -> (w1064:dbl)
        n674 = local read "Reading Value 2"() -> (w1062:dbl)
        n675 = local read "Reading Value 3"() -> (w1060:dbl)
        n676 = local read "Reading Value 4"() -> (w1058:dbl)
        n677 = local read "Reading Value 5"() -> (w1056:dbl)
        n678 = local read "Cal Value 1"() -> (w1063:dbl)
        n679 = local read "Cal Value 2"() -> (w1061:dbl)
        n680 = local read "Cal Value 3"() -> (w1059:dbl)
        n681 = local read "Cal Value 4"() -> (w1057:dbl)
        n682 = local read "Cal Value 5"() -> (w1055:dbl)
        n683 = local read "a0"() -> (w1054:dbl)
        n684 = local read "a1"() -> (w1053:dbl)
        n685 = local read "a2"() -> (w1052:dbl)
        n686 = local read "a3"() -> (w1051:dbl)
        n687 = local read "a4"() -> (w1050:dbl)
        n688 = Build Array(w1064, w1063, w1062, w1061, w1060, w1059, w1058, w1057, w1056, w1055, w1054, w1053, w1052, w1051, w1050) -> (w1109:dbl[])
        n689 = Format Into String(w1079) -> (resulting string=w1075:string)  [unwired: 3 in, 1 out]
        n690 = Format Into String(w1080) -> (resulting string=w1072:string)  [unwired: 3 in, 1 out]
        n691 = Index Array(array=w1067, index (col) #1=0 ("disabled index (col)"), index (col) #2=1 ("index (col)")) -> (element #1=w1076:string[], element #2=w1074:string[])  [unwired: 2 in]
        n692 = Search 1D Array(1D array=w1076, element=w1075) -> (index of element=w1073:i32)  [unwired: 1 in]
        n693 = disable-structure shown="Enabled" {
          disable-tunnel: w1074 -> [w1116 _]
          disable-tunnel: w1073 -> [w1115 w1117]
          disable-tunnel: w1072 -> [w1114 _]
          disable-tunnel: [w1113 w1117] -> w1066
          frame Disabled {
            n694 = Search 1D Array(1D array=w1116, element=w1114, start index (0)=w1115) -> (index of element=w1113:i32)
          }
          frame Enabled {
          }
        }
        n695 = Index Array(array=w1082, index (col) #1=0 ("disabled index (col)"), index (col) #2=1 ("disabled index (col)")) -> (element #1=w1086:string[], element #2=w1085:string[])  [unwired: 2 in]
        n696 = Format Date/Time String(time format string (%c)="%d%b%y %I:%M:%S %p") -> (date/time string=w1107:string)  [unwired: 2 in]
        n697 = Interleave 1D Arrays(w1086, w1085) -> (w1084:string[])
        n698 = Index Array(array=w1067, index (row)=w1066) -> (element=w1065:string[])  [unwired: 1 in]
        n699 = To Upper Case(1:w1107) -> (0:w1069:string)
        n700 = case shown="True" w1070 {
          tunnel: w1109 -> [w1121 _]
          tunnel: [w1119 w1123] -> w1108
          tunnel: [w1118 w1122] -> w1068
          tunnel: w1069 -> [w1118 _]
          tunnel: w1065 -> [_ w1125]
          frame False {
            n701 = Number To Fractional String(number=w1121, precision (6)=i16 16) -> (F-format string=w1119:string[])  [unwired: 2 in]
          }
          frame True {
            n702 = Array Subset(array=w1125, index=2, length=9) -> (w1123:string[])
            n703 = Index Array(array=w1125, index=11) -> (element=w1122:string)
          }
        }
        n704 = Build Array (concatenate)(w1075, w1072, w1108, w1068, w1084) -> (w1105:string[])
        n705 = Greater?(x=w1066, y=w1096) -> (0:w1095:bool)
        n706 = Subtract(x=w1066, y=w1096) -> (x-y=w1094:i32)
        n707 = Bundle(cluster=T12 {"Row"=0, "Column"=0} ("Active Cell:Active Cell"), "Row"=w1066, "Column"=-2) -> (w1097:T12)
        n708 = Select(t=w1094, s=w1095, f=u16 0 ("y")) -> (s? t:f=w1091:i32)
        n709 = Replace Array Subset(array=w1067, new element=w1105, index (row)=w1066) -> (w1102:string[][])  [unwired: 1 in]
        n710 = Bundle(cluster=T12 {"Row"=0, "Column"=0} ("Active Cell:Active Cell"), "Row"=w1091, "Column"=0) -> (w1090:T12)
        n711 = Build Array (concatenate)(w1103, w1102) -> (w1101:string[][])
        n712 = Insert Into Array(array=w1110, index=0, new element=string[] ["Write to Excel", "Load Cal File", "Cal Review Prep"]) -> (w1111:string[])
        n713 = property on="Cal Table" class="Tbl (strict)"("Active Cell"=w1097, "Cell BG Color"=u32 16775793, "Index Values"=w1090) -> ()  [unwired: 2 in, 2 out]
        n714 = call-poly <vilib>:"Write To Spreadsheet File.vi"("delimiter (\\t)"="," ("delimiter (\\t)"), "2D data"=w1101, "file path (dialog if empty)"=w1081) -> ()  [unwired: 5 in, 1 out]
      }
      frame "Distribute Calibration" {
        # "have to add in waiting screen, reread on main program, switch to streaming calibrated data and verification for that"
        n715 = Unbundle By Name(w1133) -> ("Desired System.ID"=w1130:string, "Cal File Path"=w1135:path)
        n716 = Concatenate Strings("192.168.1." ("string"), w1130) -> (w1131:string)
        n717 = Format Into String(format string="%s.cal", w1130) -> (resulting string=w1132:string)  [unwired: 2 in, 1 out]
        n718 = flat-sequence {
          tunnel: w1131 -> [w1140]
          tunnel: w1132 -> [w1139]
          tunnel: w1135 -> [w1138]
          frame #0 {
            n719 = call <vilib>:"FTP Put File.vi"("password"="", "user"="anonymous", "local path"=w1138, "remote path"=w1139, "host"=w1140) -> ()  [unwired: 5 in, 2 out]
          }
        }
      }
      frame "Calc Dev" {
        n720 = Unbundle By Name(w1148) -> ("Verify Table"=w1145:string[][], "Cal Unit"=w1143:T1, "Rack Version"=w1142:T8, "Verify Table Ref"=w1141:refnum<vi>)
        n721 = call "Calc Dev (DAQ Rack).vi"("Verify Table IN"=w1145, "Units"=w1143, "Rack Version"=w1142, "Dev Table 1 Ref"=w1141) -> ("Verify Table OUT"=w1144:string[][])  [unwired: 15 in]
        n722 = local write "Verify Table"(w1144) -> ()
        n723 = Bundle By Name(cluster=w1148, "Verify Table"=w1144) -> (w1147:T9)
        n724 = Insert Into Array(array=w1150, index=0, new element=string[] []) -> (w1149:string[])
      }
      frame "Write to Excel" {
        # "DID NOT FORMAT EXCEL FOR CDAQ"
        n725 = Unbundle By Name(w1159) -> ("Cal Spreadsheet Path"=w1163:path, "Verify Table"=w1156:string[][], "Channel to Cal"=w1153:T2, "Cal Unit"=w1152:T1)
        n726 = flat-sequence {
          tunnel: w1163 -> [w1170]
          tunnel: [w1170] -> w1164
          tunnel: [w1167] -> w1157
          tunnel: w1156 -> [w1167]
          tunnel: [w1166] -> w1155
          tunnel: w1153 -> [w1166]
          tunnel: [w1165] -> w1154
          tunnel: w1152 -> [w1165]
          tunnel: w1164 -> [w1174]
          tunnel: w1157 -> [w1173]
          tunnel: w1155 -> [w1172]
          tunnel: w1154 -> [w1171]
          frame #0 {
            n727 = property on="Main Tab" class="TabCtl (strict)"("DisabledEnum"=T10."Disabled" ("Disabled")) -> ()  [unwired: 2 in, 2 out]
            n728 = property on="Load Indicator Tab" class="TabCtl (strict)"("Visible"=TRUE) -> ()  [unwired: 2 in, 2 out]
          }
          frame #1 {
            n729 = call "cDAQ Write Data.vi"("Cal Unit"=w1171, "Channel to Cal"=w1172, "Verify Table"=w1173, "Cal Path"=w1174) -> ()  [unwired: 8 in]
          }
          frame #2 {
            n730 = property on="Main Tab" class="TabCtl (strict)"("DisabledEnum"=T10."Enabled" ("Disabled")) -> ()  [unwired: 2 in, 2 out]
            n731 = property on="Load Indicator Tab" class="TabCtl (strict)"("Visible"=FALSE) -> ()  [unwired: 2 in, 2 out]
          }
        }
        n732 = Insert Into Array(array=w1161, index=0, new element=string[] ["Recolor Tables"]) -> (w1160:string[])
      }
      frame "Recolor Tables" {
        n733 = Unbundle By Name(w1181) -> ("Verify Table Ref"=w1180:refnum<vi>)
        n734 = property on="Property Node" class="Tbl (strict)"(reference=w1180, "Active Cell"=T12 {"Row"=-2, "Column"=-2} ("Active Cell:Active Cell"), "Cell BG Color"=u32 15527148) -> (reference out=w1177:refnum<vi>)  [unwired: 1 in, 1 out]
        n735 = property on="Property Node" class="Tbl (strict)"(reference=w1177, "Active Cell"=T12 {"Row"=-2, "Column"=1} ("Active Cell:Active Cell"), "Cell BG Color"=u32 16448250) -> ()  [unwired: 1 in, 2 out]
      }
      frame "End Cal" {
        w1186 = FALSE ("1st Point Cal")
        w1185 = T10."Disabled and Grayed Out" ("Disabled")
        w1189 = 0.0 ("Reading Value 1")
        w1193 = FALSE ("Visible")
        n736 = disable-structure shown="Disabled" {
          frame Disabled {
            n737 = property on="Cancel Verify" class="Bool"("Value"=FALSE ("Cancel Cal")) -> ()  [unwired: 2 in, 2 out]
          }
          frame Enabled {
          }
        }
        n738 = property on="Output Tab" class="TabCtl (strict)"("Visible"=w1193) -> ()  [unwired: 2 in, 2 out]
        n739 = property on="Header Tab" class="TabCtl (strict)"("Visible"=w1193) -> ()  [unwired: 2 in, 2 out]
        n740 = property on="Load Indicator Tab" class="TabCtl (strict)"("Visible"=w1193) -> ()  [unwired: 2 in, 2 out]
        n741 = property on="Main Tab" class="TabCtl (strict)"("DisabledEnum"=T10."Enabled" ("Disabled")) -> ()  [unwired: 2 in, 2 out]
        n742 = property on="Header" class="Bool"("DisabledEnum"=T10."Enabled" ("Disabled")) -> ()  [unwired: 2 in, 2 out]
        n743 = local write "Reading Value 1"(w1189) -> ()
        n744 = local write "Cal Value 1"(w1189) -> ()
        n745 = local write "Reading Value 2"(w1189) -> ()
        n746 = local write "Cal Value 2"(w1189) -> ()
        n747 = local write "Reading Value 3"(w1189) -> ()
        n748 = local write "Cal Value 3"(w1189) -> ()
        n749 = local write "Reading Value 4"(w1189) -> ()
        n750 = local write "Cal Value 4"(w1189) -> ()
        n751 = local write "Reading Value 5"(w1189) -> ()
        n752 = local write "Cal Value 5"(w1189) -> ()
        n753 = local write "a0"(w1189) -> ()
        n754 = local write "a1"(w1189) -> ()
        n755 = local write "a2"(w1189) -> ()
        n756 = local write "a3"(w1189) -> ()
        n757 = local write "a4"(w1189) -> ()
        n758 = property on="Start Cal" class="Bool"("DisabledEnum"=w1185) -> ()  [unwired: 2 in, 2 out]
        n759 = property on="Channel to Cal" class="Enum (strict)"("DisabledEnum"=w1185) -> ()  [unwired: 2 in, 2 out]
        n760 = property on="View Spreadsheet" class="Bool"("DisabledEnum"=w1185) -> ()  [unwired: 2 in, 2 out]
        n761 = property on="Start Verification" class="Bool"("DisabledEnum"=w1185) -> ()  [unwired: 2 in, 2 out]
        n762 = local write "RIO Found"(FALSE ("RIO Found")) -> ()
        n763 = local write "Tank IP:"("" ("Tank IP:")) -> ()
        n764 = call "TCP Data Stream PC.vi"("Mode"=TCP_Data_Stream_Mode_(PC)."Close") -> ()  [unwired: 15 in, 4 out]
        n765 = disable-structure shown="Disabled" {
          disable-tunnel: w1185 -> [w1199 _]
          frame Disabled {
            n766 = property on="Cal Unit" class="Enum (strict)"("DisabledEnum"=w1199) -> ()  [unwired: 2 in, 2 out]
          }
          frame Enabled {
          }
        }
        n767 = local write "1st Point Cal"(w1186) -> ()
        n768 = local write "2nd Point Cal"(w1186) -> ()
        n769 = local write "3rd Point Cal"(w1186) -> ()
        n770 = local write "4th Point Cal"(w1186) -> ()
        n771 = local write "5th Point Cal"(w1186) -> ()
        n772 = Insert Into Array(array=w1197, index=0, new element=string[] ["Recolor Tables", "Init Cal"]) -> (w1198:string[])
      }
      frame "Increment Channel" {
        n773 = Unbundle By Name(w1203) -> ("Channel to Cal"=w1202:T2)
        n774 = Increment(x=w1202) -> (x+1=w1201:T2)
        n775 = Bundle By Name(cluster=w1203, "Channel to Cal"=w1201) -> (w1204:T9)
        n776 = local write "Channel to Cal"(w1201) -> ()
      }
      frame "Exit" {
        n777 = local write "Stop Second Loop"(TRUE ("Stop Second Loop")) -> ()
      }
    }
  }
  n778 = while {
    tunnel: w3 -> [_]
    shift-right: [w1210] -> _
    shift-left: _ -> [w1211]
    stop <- "Stop Second Loop" stop-if-true
    n779 = local read "Channel to Cal"() -> (w1209:T2)
    n780 = local read "RIO Found"() -> (w1214:bool)
    n781 = Wait (ms)(milliseconds to wait=u32 10) -> ()  [unwired: 1 out]
    n782 = case shown="True" w1214 {
      tunnel: w1209 -> [_ w1217]
      tunnel: [0.0 ("Data Out") w1222] -> w1210
      tunnel: w1211 -> [_ w1221]
      frame False {
        n783 = Wait (ms)(milliseconds to wait=u32 500) -> ()  [unwired: 1 out]
      }
      frame True {
        n784 = call "cDAQ AI Read.vi"("Channel to Cal"=w1217) -> ("Lost Connection"=→"Lost Connection":bool, "Available?"=w1219:bool, "Data"=w1218:dbl)  [unwired: 8 in]
        n785 = case shown="True" w1219 {
          tunnel: w1218 -> [_ w1225]
          tunnel: [w1223 w1224] -> w1222
          tunnel: w1221 -> [w1223 _]
          frame False {
          }
          frame True {
            n786 = call <vilib>:"Mean PtByPt.vi"("x"=w1225, "sample length"="avg") -> ("mean"=w1224:dbl)  [unwired: 2 in, 1 out]
          }
        }
      }
    }
    "Cal Reading" <- w1210
    "Ver Reading" <- w1210
  }
